vi "Multiple Class_Multiple State_Block Chain.vi"() -> ()   [LabVIEW 2021]
uses:
  Commander/Commander.lvclass
  C:/Program Files (x86)/Hyper State Machine Framework/SSW_Hyper_State_Machine.lvlibp/State_Machine_Class/Main_State_Machine/Hyper_State_Machine.lvclass
  C:/Program Files (x86)/Hyper State Machine Framework/SSW_Hyper_State_Machine.lvlibp/State_Interface/State_Interface.lvclass
  Common_State/Common_State.lvclass
  Image_Acquisition/Image_Acquisition.lvclass
  Motion_Control/Motion_Control.lvclass
  Data_Logging/Data_Logging.lvclass
  DIO/DIO.lvclass
  C:/Program Files (x86)/Hyper State Machine Framework/SSW_Hyper_State_Machine.lvlibp/State_Machine_Class/State_Machine_Module.llb/State Machine.ctl
  C:/Program Files (x86)/Hyper State Machine Framework/SSW_Hyper_State_Machine.lvlibp/State_Machine_Class/State_Machine_Module.llb/Lock_Unlock.ctl
  C:/Program Files (x86)/Hyper State Machine Framework/SSW_Hyper_State_Machine.lvlibp/State_Machine_Class/State_Machine_Module.llb/Iterval.ctl
  C:/Program Files (x86)/Hyper State Machine Framework/SSW_Hyper_State_Machine.lvlibp/State_Machine_Class/State_Machine_Module.llb/Time_Out.ctl
  <vilib>/numeric/Random Number (Range) DBL.vi
  <vilib>/Utility/High Resolution Relative Seconds.vi
  C:/Program Files (x86)/Hyper State Machine Framework/SSW_Hyper_State_Machine.lvlibp
panel:
  out "Child_State#":u32
  out "Activate":bool
  out "Lamp":bool
  out "Current_Pos":dbl caption="mm"
  in  "EMO":bool
  out "Product ID":string
  in  "Activate_Code(Blank for 30 min Trial)":string="ROeInPkJ3DxAXwEgzbbW2XA0t1jaS1URlS9jikesQMED6VfU"
  out "Heart_Rate":bool
  out "Heart rate(s)":dbl format="%#_6p"
  out "Execute rate(Hz)":dbl format="%#_6p"
  out "Base Class_Time_Act":bool
  out "Base Class_Elapsed Time(s)":dbl format="%#_6p"
  out "Base Class":bool=TRUE
  out "Base Class_Remaining(s)":dbl format="%#_6p"
  out "Base Class Progress":dbl(slide) scale=0.0..10.0
  in  "Base Class":dbl=10.0 max=1000.0 format="%#_13p"
  out "Base Class":string
  out "Base Class_Active":bool
  in  "Action Manager":T1(ring)
  out "Common":bool=TRUE
  out "Common_State":string
  out "Common_Time_Act":bool
  out "Common_Elapsed Time(s)":dbl format="%#_6p"
  out "Common_State Progress":dbl(slide) scale=0.0..5.0
  in  "Common_State_Interval":dbl=5.0 max=1000.0 format="%#_13p"
  out "Common_State_Active":bool
  out "Common_State_Remaining(s)":dbl format="%#_6p"
  out "Data Logging Progress":dbl(slide) scale=0.0..3.0
  out "DIO Progress":dbl(slide) scale=0.0..0.01
  out "Motion Control Progress":dbl(slide) scale=0.0..0.5
  out "Image Acquisition Progress":dbl(slide) scale=0.0..0.01
  out "Commander Progress":dbl(slide)=-1.0 scale=0.0..1.0
  out "Data_Logging":bool=TRUE
  out "Data Logging":string
  out "Data_Logging_Time_Act":bool
  out "Data_Logging_Elapsed Time(s)":dbl format="%#_6p"
  out "DIO":bool=TRUE
  out "DIO":string
  out "DIO_Time_Act":bool
  out "DIO_Elapsed Time(s)":dbl format="%#_6p"
  out "Motion_Control":bool=TRUE
  out "Motion_Control":string
  out "Motion_Control_Time_Act":bool
  out "Motion_Control_Elapsed Time(s)":dbl format="%#_6p"
  in  "Data Logging":dbl=3.0 max=1000.0 format="%#_13p"
  out "Data Logging_Active":bool
  out "Data Logging_Remaining(s)":dbl format="%#_6p"
  in  "DIO_Interval":dbl=0.01 max=1000.0 format="%#_13p"
  in  "Motion_Control_Interval":dbl=0.5 max=1000.0 format="%#_13p"
  out "Motion Control_Act":bool
  out "DIO_Act":bool
  out "DIO_Remaining(s)":dbl format="%#_6p"
  out "Motion_Control_Remaining(s)":dbl format="%#_6p"
  in  "Image Acquisition_Interval":dbl=0.01 max=1000.0 format="%#_13p"
  in  "Commander_Interval":dbl max=1000.0 format="%#_13p"
  in  "System_Wait_Time":dbl=0.025 format="%#_13p"
  out "Commander_Active":bool
  out "Image Acquisition_Act":bool
  out "Image Acquisition_Remaining(s)":dbl format="%#_6p"
  out "Commander_Remaining(s)":dbl format="%#_6p"
  out "Image Acquisition":bool=TRUE
  out "Image Acquisition":string
  out "Commander":bool=TRUE
  out "Image Acquisition_Time_Act":bool
  out "Image Acquisition_Elapsed Time(s)":dbl format="%#_6p"
  out "Commander":string
  out "State1_Time_Act":bool
  out "Commander_Elapsed Time(s)":dbl format="%#_6p"
  in  "Stop":bool
  # "Note : Each State is Waiting Until Commader State Finished on \"Interval_Delay\" and then Unlock"
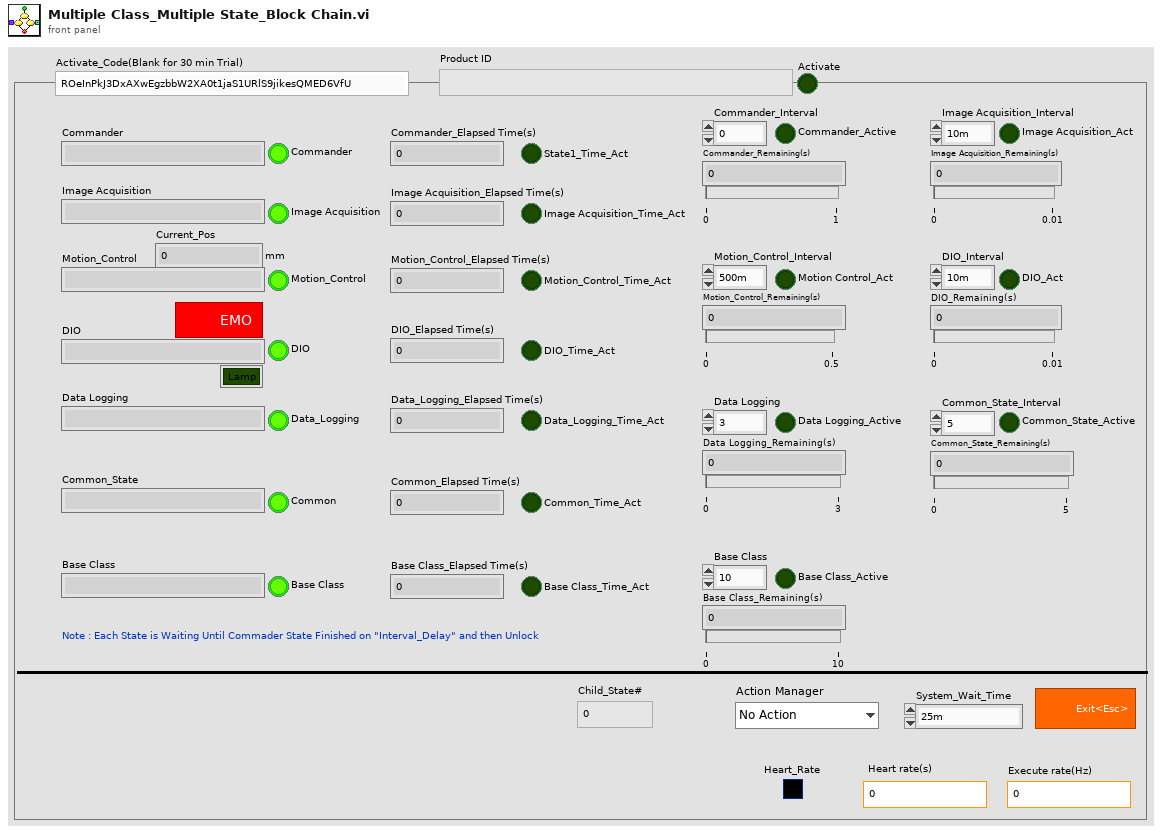
[diagram p1: front panel]
types:
  T1 = enum16{"No Action", "Init", "Lock", "Unlock", "Release"}
  T2 = typedef "SSW_Hyper_State_Machine.lvlibp/State Machine.ctl" = cluster{"Command":string, "Data":variant}
  T3 = typedef "SSW_Hyper_State_Machine.lvlibp/Time_Out.ctl" = cluster{"Enable(True)":bool, "Time Out_State Name":string, "Time Target (1s)":dbl, "Time Out_Reply Message_State":string}
  T4 = typedef "SSW_Hyper_State_Machine.lvlibp/Lock_Unlock.ctl" = cluster{"Action_Mode (Get)":enum16{"Set", "Get"}, "Action_Set (False)":bool, "State_In (Wait)":string}
  T5 = typedef "SSW_Hyper_State_Machine.lvlibp/Iterval.ctl" = cluster{"Delay(s)":dbl, "State (Interval_Delay)":string}
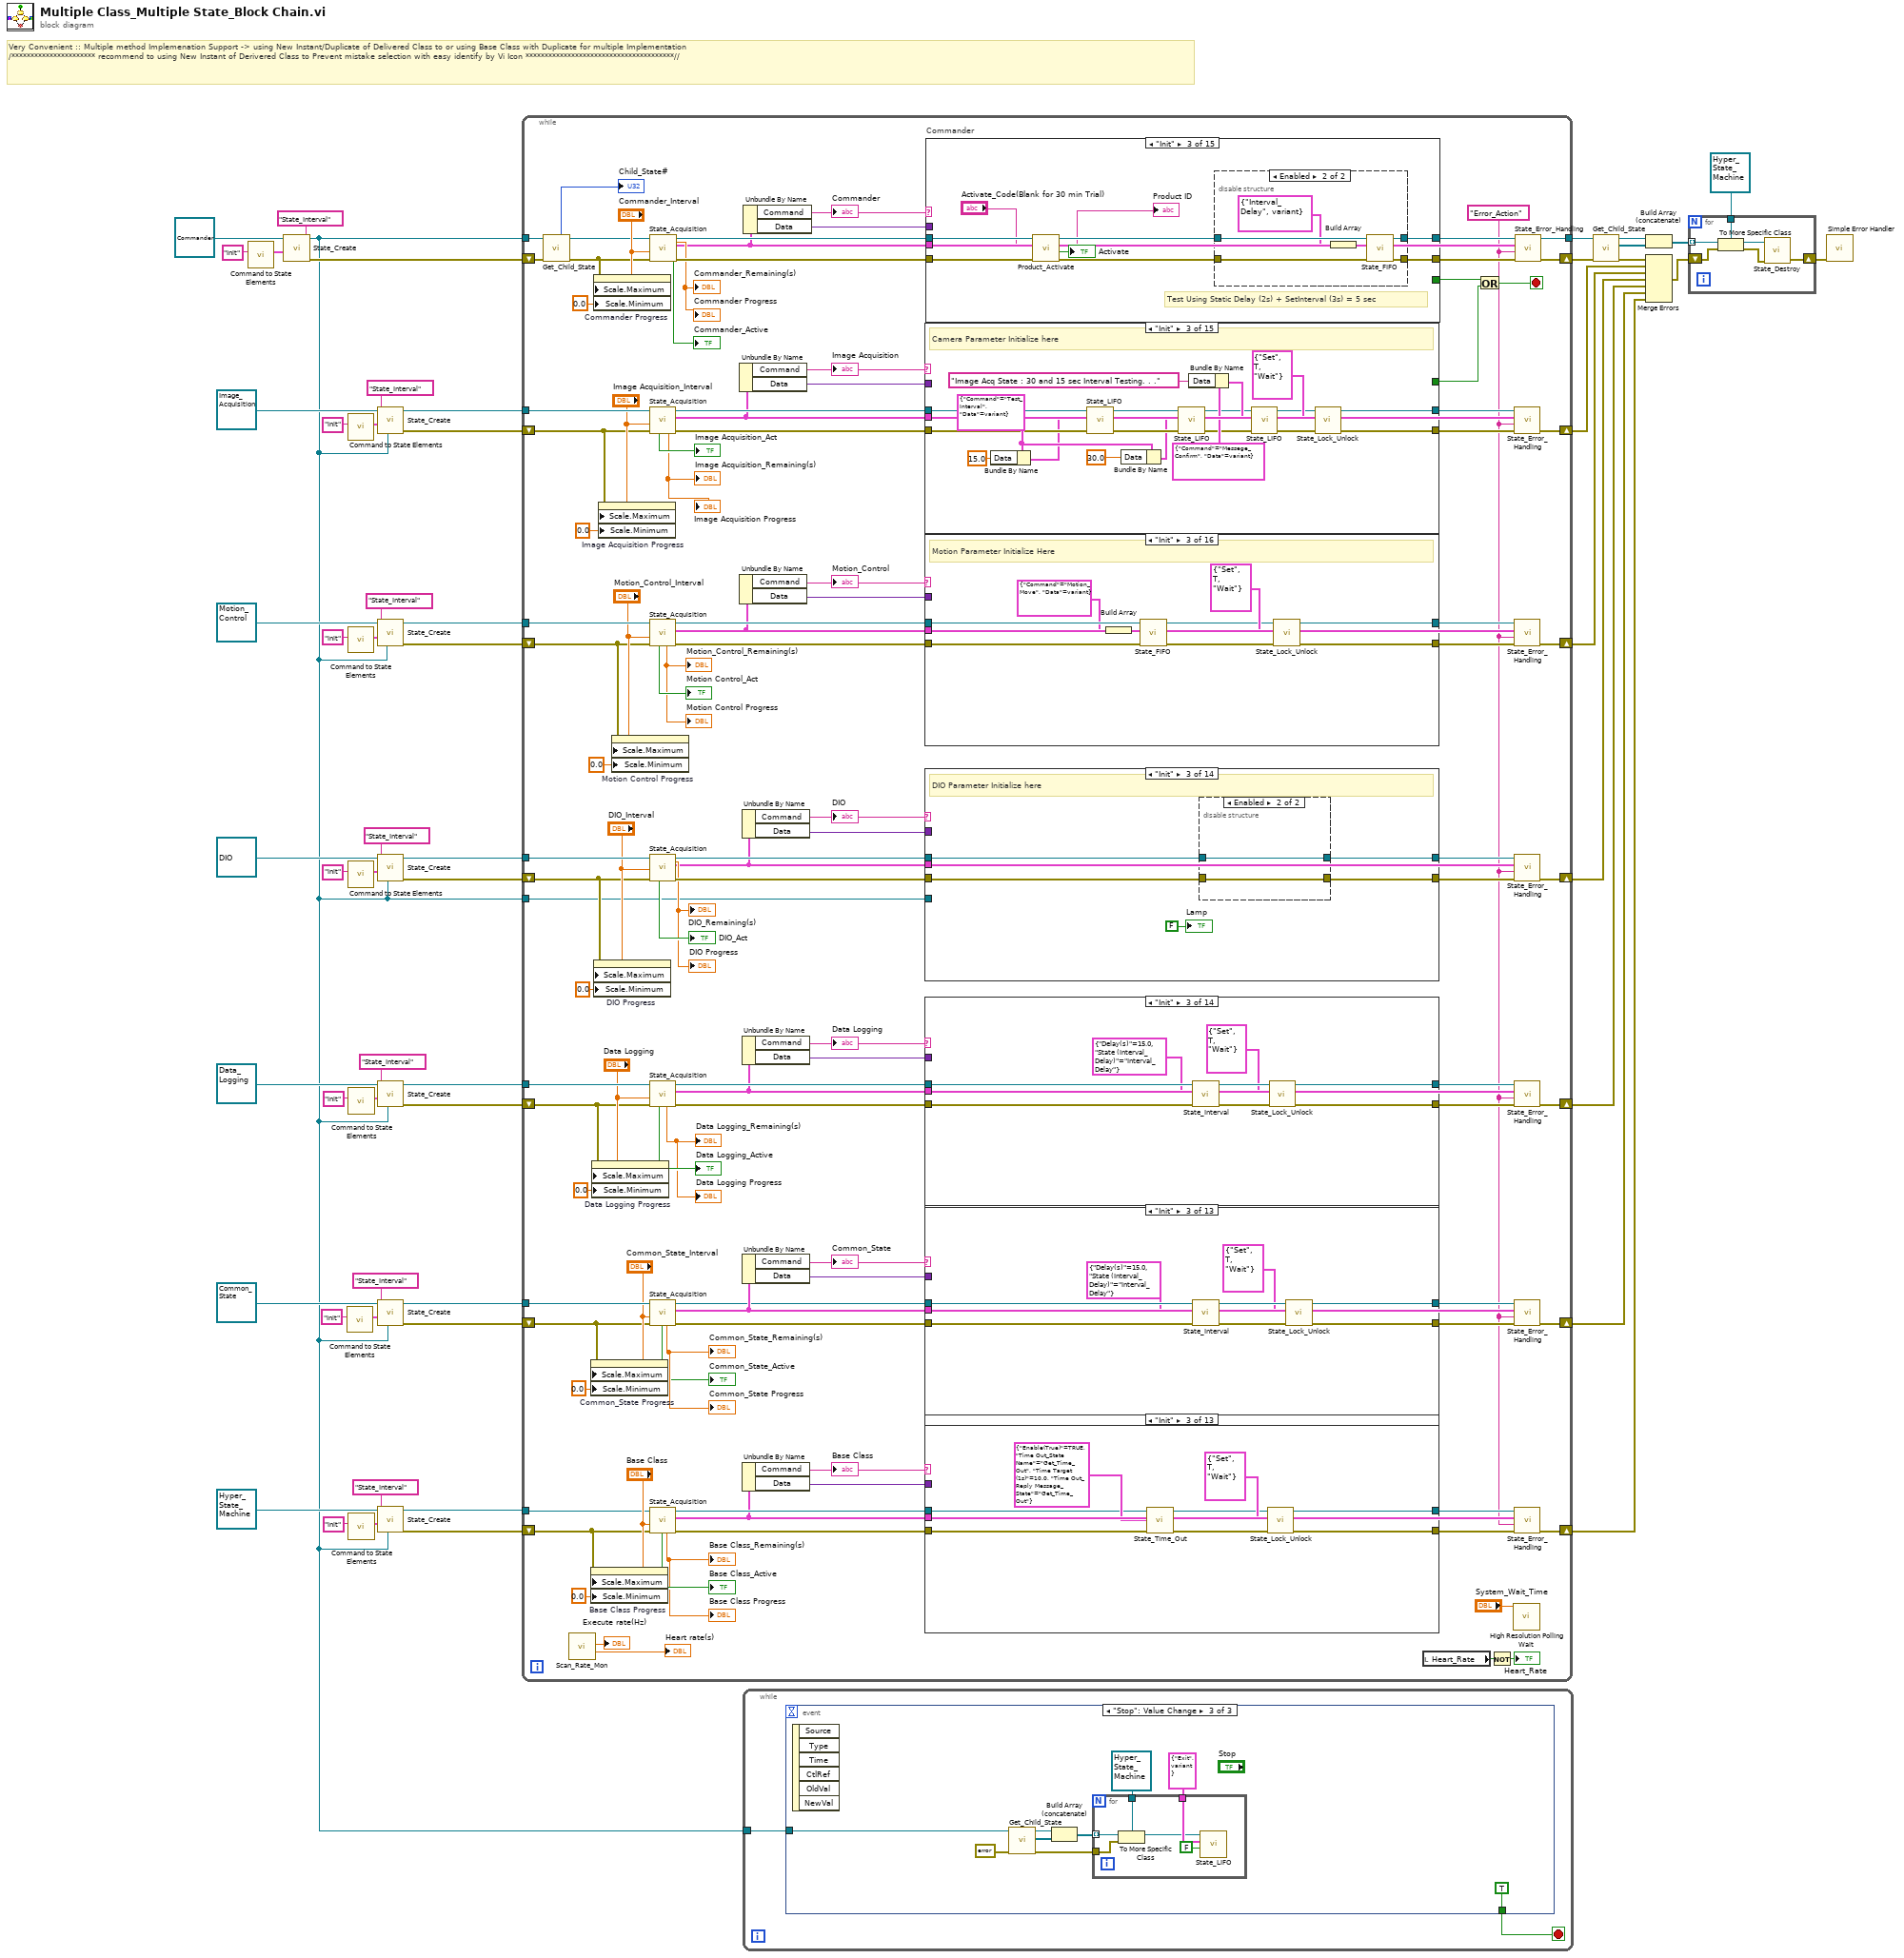
[diagram p0: block diagram]
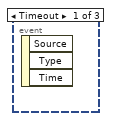
[diagram p2: hidden frame]
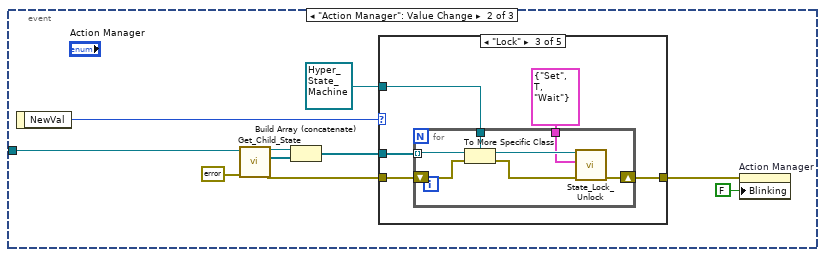
[diagram p3: hidden frame]
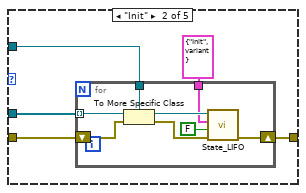
[diagram p5: hidden frame]
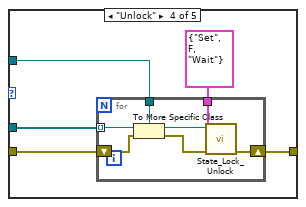
[diagram p6: hidden frame]
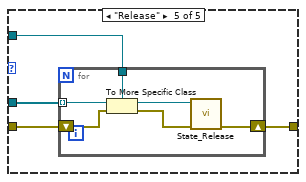
[diagram p7: hidden frame]
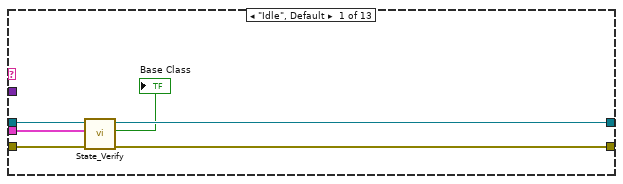
[diagram p8: hidden frame]
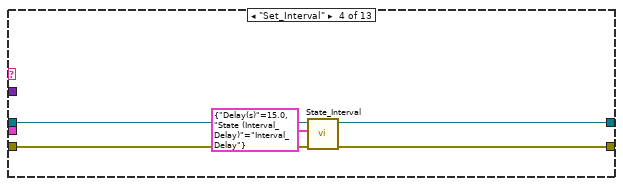
[diagram p10: hidden frame]
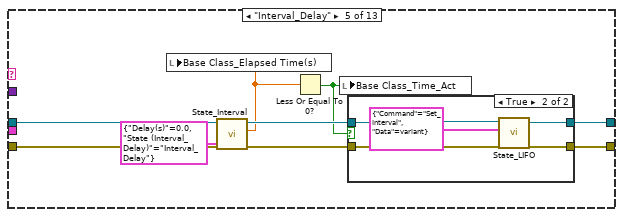
[diagram p11: hidden frame]
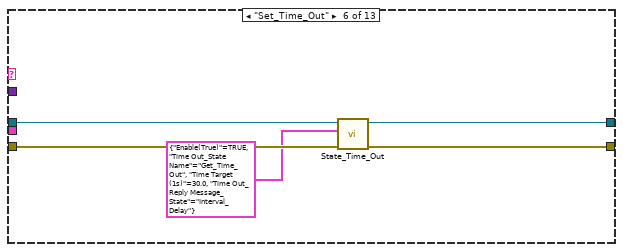
[diagram p13: hidden frame]
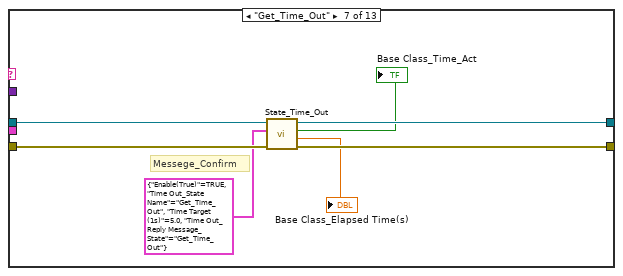
[diagram p14: hidden frame]
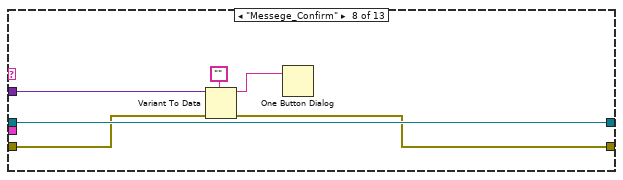
[diagram p15: hidden frame]
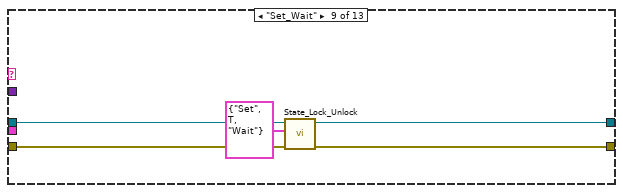
[diagram p16: hidden frame]
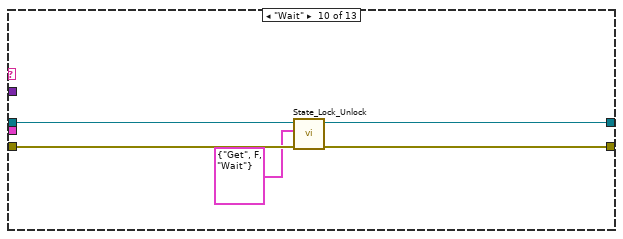
[diagram p17: hidden frame]
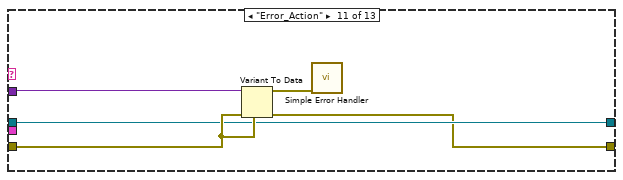
[diagram p18: hidden frame]
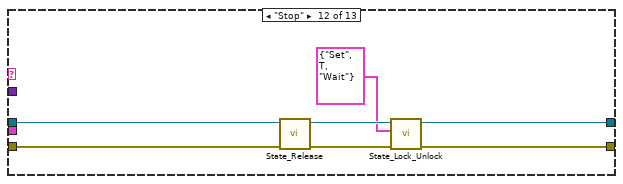
[diagram p19: hidden frame]
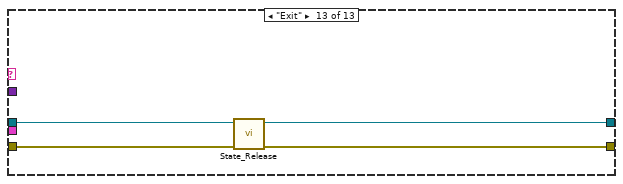
[diagram p20: hidden frame]
diagram:
  # "Very Convenient :: Multiple method Implemenation Support -> using New Instant/Duplicate of Delivered Class to or using Base Class with Duplicate for multiple Implementation\n/********************** recommend to using New Instant of Derivered Class to Prevent mistake selection with easy identify by Vi Icon ***************************************//"
  n1 = call "Command to State Elements.vi"("Command"="Init") -> ("Command to State Elements"=w40:T2)  [unwired: 10 in]
  n2 = call-dynamic "State_Create.vi"("Init_State(Option)"=w40, "State_Interval_Name"="State_Interval" ("Core_Interval_Name(State_Interval)"), "State_Machine_Class in"=refnum<class "Commander.lvclass"> refnum ("Commander.lvclass")) -> ("error out"=w57:errorcluster, "State_Machine_Class out"=w16:refnum<class "Commander.lvclass">)  [unwired: 6 in, 1 out]
  n3 = call "Command to State Elements.vi"("Command"="Init") -> ("Command to State Elements"=w32:T2)  [unwired: 10 in]
  n4 = call "Command to State Elements.vi"("Command"="Init") -> ("Command to State Elements"=w42:T2)  [unwired: 10 in]
  n5 = call "Command to State Elements.vi"("Command"="Init") -> ("Command to State Elements"=w38:T2)  [unwired: 10 in]
  n6 = call "Command to State Elements.vi"("Command"="Init") -> ("Command to State Elements"=w36:T2)  [unwired: 10 in]
  n7 = call "Command to State Elements.vi"("Command"="Init") -> ("Command to State Elements"=w34:T2)  [unwired: 10 in]
  n8 = call "Command to State Elements.vi"("Command"="Init") -> ("Command to State Elements"=w30:T2)  [unwired: 10 in]
  n9 = call-dynamic "State_Create.vi"("Block_Chain"=w16, "Init_State(Option)"=w42, "State_Interval_Name"="State_Interval" ("Core_Interval_Name(State_Interval)"), "State_Machine_Class in"=refnum<class "Image_Acquisition.lvclass"> refnum ("Image_Acquisition.lvclass")) -> ("error out"=w56:errorcluster, "State_Machine_Class out"=w22:refnum<class "Image_Acquisition.lvclass">)  [unwired: 5 in, 1 out]
  n10 = call-dynamic "State_Create.vi"("Block_Chain"=w16, "Init_State(Option)"=w38, "State_Interval_Name"="State_Interval" ("Core_Interval_Name(State_Interval)"), "State_Machine_Class in"=refnum<class "Motion_Control.lvclass"> refnum ("Motion_Control.lvclass")) -> ("error out"=w51:errorcluster, "State_Machine_Class out"=w21:refnum<class "Motion_Control.lvclass">)  [unwired: 5 in, 1 out]
  n11 = call-dynamic "State_Create.vi"("Block_Chain"=w16, "Init_State(Option)"=w36, "State_Interval_Name"="State_Interval" ("Core_Interval_Name(State_Interval)"), "State_Machine_Class in"=refnum<class "DIO.lvclass"> refnum ("DIO.lvclass")) -> ("error out"=w50:errorcluster, "State_Machine_Class out"=w20:refnum<class "DIO.lvclass">)  [unwired: 5 in, 1 out]
  n12 = call-dynamic "State_Create.vi"("Block_Chain"=w16, "Init_State(Option)"=w34, "State_Interval_Name"="State_Interval" ("Core_Interval_Name(State_Interval)"), "State_Machine_Class in"=refnum<class "Data_Logging.lvclass"> refnum ("Data_Logging.lvclass")) -> ("error out"=w49:errorcluster, "State_Machine_Class out"=w19:refnum<class "Data_Logging.lvclass">)  [unwired: 5 in, 1 out]
  n13 = call-dynamic "State_Create.vi"("Block_Chain"=w16, "Init_State(Option)"=w32, "State_Interval_Name"="State_Interval" ("Core_Interval_Name(State_Interval)"), "State_Machine_Class in"=refnum<class "Common_State.lvclass"> refnum ("Common_State.lvclass")) -> ("error out"=w47:errorcluster, "State_Machine_Class out"=w18:refnum<class "Common_State.lvclass">)  [unwired: 5 in, 1 out]
  n14 = call-dynamic "State_Create.vi"("Parent_State"=w16, "Init_State(Option)"=w30, "State_Interval_Name"="State_Interval" ("Core_Interval_Name(State_Interval)"), "State_Machine_Class in"=refnum<class "Hyper_State_Machine.lvclass"> refnum ("SSW_Hyper_State_Machine.lvlibp:Hyper_State_Machine.lvclass")) -> ("error out"=w44:errorcluster, "State_Machine_Class out"=w17:refnum<class "Hyper_State_Machine.lvclass">)  [unwired: 5 in, 1 out]
  n15 = while {
    tunnel: w16 -> [w62]
    shift-right: [w163] -> w14
    shift-left: w57 -> [w61]
    tunnel: [w162] -> w15
    tunnel: w22 -> [w158]
    shift-right: [w157] -> w6
    shift-left: w56 -> [w69]
    tunnel: w21 -> [w134]
    tunnel: w20 -> [w133]
    tunnel: w19 -> [w132]
    shift-right: [w131] -> w5
    shift-left: w51 -> [w68]
    shift-right: [w130] -> w4
    shift-left: w50 -> [w67]
    shift-right: [w129] -> w3
    shift-left: w49 -> [w66]
    tunnel: w18 -> [w108]
    shift-right: [w107] -> w2
    shift-left: w47 -> [w65]
    shift-right: [w77] -> w1
    shift-left: w44 -> [w64]
    tunnel: w17 -> [w81]
    tunnel: w16 -> [w63]
    stop <- w155 stop-if-true
    w76 = "Error_Action" ("State_Error_Handling")
    n16 = call-dynamic "Get_Child_State.vi"("error in (no error)"=w61, "Hyper_State_Machine in"=w62) -> ("error out"=w60:errorcluster, "Hyper_State_Machine out"=w59:refnum<class "Commander.lvclass">, "Child_State#"=→"Child_State#":u32)  [unwired: 5 in, 2 out]
    n17 = call "Scan_Rate_Mon.vi"() -> ("Heart rate(s)"=→"Heart rate(s)":dbl, "Execute rate(Hz)"=→"Execute rate(Hz)":dbl)
    n18 = property on="Common_State Progress" class="Slide (strict)"(error in=w65, "Scale.Maximum"="Common_State_Interval", "Scale.Minimum"=0.0 ("Scale.Range:Minimum")) -> ()  [unwired: 1 in, 2 out]
    n19 = property on="Base Class Progress" class="Slide (strict)"(error in=w64, "Scale.Maximum"="Base Class", "Scale.Minimum"=0.0 ("Scale.Range:Minimum")) -> ()  [unwired: 1 in, 2 out]
    n20 = property on="Data Logging Progress" class="Slide (strict)"(error in=w66, "Scale.Maximum"="Data Logging", "Scale.Minimum"=0.0 ("Scale.Range:Minimum")) -> ()  [unwired: 1 in, 2 out]
    n21 = property on="Commander Progress" class="Slide (strict)"(error in=w60, "Scale.Maximum"="Commander_Interval", "Scale.Minimum"=0.0 ("Scale.Range:Minimum")) -> ()  [unwired: 1 in, 2 out]
    n22 = property on="DIO Progress" class="Slide (strict)"(error in=w67, "Scale.Maximum"="DIO_Interval", "Scale.Minimum"=0.0 ("Scale.Range:Minimum")) -> ()  [unwired: 1 in, 2 out]
    n23 = property on="Image Acquisition Progress" class="Slide (strict)"(error in=w69, "Scale.Maximum"="Image Acquisition_Interval", "Scale.Minimum"=0.0 ("Scale.Range:Minimum")) -> ()  [unwired: 1 in, 2 out]
    n24 = property on="Motion Control Progress" class="Slide (strict)"(error in=w68, "Scale.Maximum"="Motion_Control_Interval", "Scale.Minimum"=0.0 ("Scale.Range:Minimum")) -> ()  [unwired: 1 in, 2 out]
    n25 = call-dynamic "State_Acquisition.vi"("error in (no error)"=w69, "State_Interval_Time(s)"="Image Acquisition_Interval", "Main_Machine_State_Class in"=w158) -> ("error out"=w161:errorcluster, "State"=w94:T2, "Main_Machine_State_Class out"=w156:refnum<class "Image_Acquisition.lvclass">, "Remaining(ms)"=→"Image Acquisition_Remaining(s)" →"Image Acquisition Progress":dbl, "Current_State_Active"=→"Image Acquisition_Act":bool)  [unwired: 2 in, 2 out]
    n26 = call-dynamic "State_Acquisition.vi"("error in (no error)"=w68, "State_Interval_Time(s)"="Motion_Control_Interval", "Main_Machine_State_Class in"=w134) -> ("error out"=w136:errorcluster, "State"=w93:T2, "Main_Machine_State_Class out"=w137:refnum<class "Motion_Control.lvclass">, "Remaining(ms)"=→"Motion_Control_Remaining(s)" →"Motion Control Progress":dbl, "Current_State_Active"=→"Motion Control_Act":bool)  [unwired: 2 in, 2 out]
    n27 = call-dynamic "State_Acquisition.vi"("error in (no error)"=w67, "State_Interval_Time(s)"="DIO_Interval", "Main_Machine_State_Class in"=w133) -> ("error out"=w143:errorcluster, "State"=w92:T2, "Main_Machine_State_Class out"=w144:refnum<class "DIO.lvclass">, "Remaining(ms)"=→"DIO_Remaining(s)" →"DIO Progress":dbl, "Current_State_Active"=→"DIO_Act":bool)  [unwired: 2 in, 2 out]
    n28 = call-dynamic "State_Acquisition.vi"("error in (no error)"=w66, "State_Interval_Time(s)"="Data Logging", "Main_Machine_State_Class in"=w132) -> ("error out"=w145:errorcluster, "State"=w91:T2, "Main_Machine_State_Class out"=w146:refnum<class "Data_Logging.lvclass">, "Remaining(ms)"=→"Data Logging_Remaining(s)" →"Data Logging Progress":dbl, "Current_State_Active"=→"Data Logging_Active":bool)  [unwired: 2 in, 2 out]
    n29 = call-dynamic "State_Acquisition.vi"("error in (no error)"=w65, "State_Interval_Time(s)"="Common_State_Interval", "Main_Machine_State_Class in"=w108) -> ("error out"=w110:errorcluster, "State"=w90:T2, "Main_Machine_State_Class out"=w75:refnum<class "Common_State.lvclass">, "Remaining(ms)"=→"Common_State_Remaining(s)" →"Common_State Progress":dbl, "Current_State_Active"=→"Common_State_Active":bool)  [unwired: 2 in, 2 out]
    n30 = call-dynamic "State_Acquisition.vi"("error in (no error)"=w64, "State_Interval_Time(s)"="Base Class", "Main_Machine_State_Class in"=w81) -> ("error out"=w82:errorcluster, "State"=w79:T2, "Main_Machine_State_Class out"=w83:refnum<class "Hyper_State_Machine.lvclass">, "Remaining(ms)"=→"Base Class_Remaining(s)" →"Base Class Progress":dbl, "Current_State_Active"=→"Base Class_Active":bool)  [unwired: 2 in, 2 out]
    n31 = call-dynamic "State_Acquisition.vi"("error in (no error)"=w60, "State_Interval_Time(s)"="Commander_Interval", "Main_Machine_State_Class in"=w59) -> ("error out"=w165:errorcluster, "State"=w95:T2, "Main_Machine_State_Class out"=w166:refnum<class "Commander.lvclass">, "Remaining(ms)"=→"Commander_Remaining(s)" →"Commander Progress":dbl, "Current_State_Active"=→"Commander_Active":bool)  [unwired: 2 in, 2 out]
    n32 = Unbundle By Name(w94) -> ("Command"=w159:string, "Data"=w160:variant)
    "Image Acquisition" <- w159
    n33 = Unbundle By Name(w93) -> ("Command"=w123:string, "Data"=w149:variant)
    "Motion_Control" <- w123
    n34 = Unbundle By Name(w92) -> ("Command"=w124:string, "Data"=w148:variant)
    "DIO" <- w124
    n35 = Unbundle By Name(w91) -> ("Command"=w125:string, "Data"=w147:variant)
    "Data Logging" <- w125
    n36 = Unbundle By Name(w90) -> ("Command"=w104:string, "Data"=w109:variant)
    "Common_State" <- w104
    n37 = Unbundle By Name(w79) -> ("Command"=w87:string, "Data"=w84:variant)
    "Base Class" <- w87
    n38 = Unbundle By Name(w95) -> ("Command"=w169:string, "Data"=w168:variant)
    "Commander" <- w169
    n39 = case shown="\"Init\"" w159 {
      selector: w159 -> [_ _ _ w659 _ _ _ _ _ _ _ _ _ _ _]
      tunnel: w160 -> [_ _ _ _ _ w674 _ _ _ w723 _ _ w737 _ _]
      tunnel: w156 -> [w635 w637 w645 w664 w669 w679 w692 w710 w717 w721 w728 w733 w734 w745 w750]
      tunnel: w161 -> [w634 w636 w640 w663 w668 w670 w691 w709 w716 w720 w727 w732 w736 w744 w749]
      tunnel: [w628 w637 w653 w662 w667 w678 w687 w708 w715 w721 w726 w731 w734 w740 w748] -> w151
      tunnel: [w627 w636 w652 w661 w666 w677 w686 w707 w714 w719 w725 w730 w735 w739 w747] -> w150
      tunnel: w94 -> [w633 _ _ _ _ _ _ _ _ _ _ _ _ _ _]
      tunnel: [_ _ _ _ _ _ _ _ _ _ _ _ _ _ TRUE] -> w154
      frame "Idle", Default {
        n40 = call-dynamic "State_Verify.vi"("error in (no error)"=w634, "State(Idle)"=w633, "State_Machine_Class in"=w635) -> ("error out"=w630:errorcluster, "Active"=→"Image Acquisition":bool, "State_Machine_Class out"=w631:refnum<class "Image_Acquisition.lvclass">)  [unwired: 6 in]
        n41 = Build Array(T2 {"Command"="Image_Acquisition", "Data"=variant} ("State")) -> (w626:T2[])
        n42 = call-dynamic "State_FIFO.vi"("error in (no error)"=w630, "State Machine[]"=w626, "State_Machine_Class in"=w631) -> ("error out"=w627:errorcluster, "State_Machine_Class out"=w628:refnum<class "Image_Acquisition.lvclass">)  [unwired: 7 in]
      }
      frame "State_Interval" {
      }
      frame "Init" {
        w648 = T2 {"Command"="Test_Interval", "Data"=variant} ("State Machine")
        # "Camera Parameter Initialize here"
        n43 = Bundle By Name(cluster=w648, "Data"=15.0) -> (w639:T2)
        n44 = call-dynamic "State_LIFO.vi"("error in (no error)"=w640, "State Machine"=w639, "State_Machine_Class in"=w645) -> ("error out"=w641:errorcluster, "State_Machine_Class out"=w644:refnum<class "Image_Acquisition.lvclass">)  [unwired: 7 in]
        n45 = Bundle By Name(cluster=w648, "Data"=30.0) -> (w638:T2)
        n46 = call-dynamic "State_LIFO.vi"("error in (no error)"=w641, "State Machine"=w638, "State_Machine_Class in"=w644) -> ("error out"=w642:errorcluster, "State_Machine_Class out"=w643:refnum<class "Image_Acquisition.lvclass">)  [unwired: 7 in]
        n47 = Bundle By Name(cluster=T2 {"Command"="Messege_Confirm", "Data"=variant} ("State Machine"), "Data"="Image Acq State : 30 and 15 sec Interval Testing. . .") -> (w650:T2)
        n48 = call-dynamic "State_LIFO.vi"("error in (no error)"=w642, "State Machine"=w650, "State_Machine_Class in"=w643) -> ("error out"=w654:errorcluster, "State_Machine_Class out"=w655:refnum<class "Image_Acquisition.lvclass">)  [unwired: 7 in]
        n49 = call-dynamic "State_Lock_Unlock.vi"("error in (no error)"=w654, "Parameter"=T4 {"Action_Mode (Get)"=enum."Set", "Action_Set (False)"=TRUE, "State_In (Wait)"="Wait"}, "State_Machine_Class in"=w655) -> ("error out"=w652:errorcluster, "State_Machine_Class out"=w653:refnum<class "Image_Acquisition.lvclass">)  [unwired: 6 in, 1 out]
      }
      frame "Image_Acquisition" {
        (unwired) T5 {"Delay(s)"=5.0, "State (Interval_Delay)"="Image_Acquisition"} ("Parameter")
        # "Simple handling with specify name"
        # "Dynamic handling Name for Waiting Demo"
        # "Image Acquisition Function Here"
        n50 = Bundle By Name(cluster=T5 {"Delay(s)"=5.0, "State (Interval_Delay)"=""} ("Parameter"), "State (Interval_Delay)"=w659) -> (w658:T5)
        n51 = call-dynamic "State_Interval.vi"("error in (no error)"=w663, "Parameter"=w658, "State_Machine_Class in"=w664) -> ("error out"=w661:errorcluster, "Elapsed Time(s)"=w657:dbl, "State_Machine_Class out"=w662:refnum<class "Image_Acquisition.lvclass">)  [unwired: 6 in]
        n52 = local write "Image Acquisition_Elapsed Time(s)"(w657) -> ()
      }
      frame "Set_Interval" {
        n53 = call-dynamic "State_Interval.vi"("error in (no error)"=w668, "Parameter"=T5 {"Delay(s)"=15.0, "State (Interval_Delay)"="Interval_Delay"}, "State_Machine_Class in"=w669) -> ("error out"=w666:errorcluster, "State_Machine_Class out"=w667:refnum<class "Image_Acquisition.lvclass">)  [unwired: 6 in, 1 out]
      }
      frame "Test_Interval" {
        n54 = Variant To Data(error in=w670, type=0.0 ("Delay(s)"), Variant=w674) -> (data=w672:dbl)  [unwired: 1 out]
        n55 = Bundle By Name(cluster=T5 {"Delay(s)"=0.0, "State (Interval_Delay)"="Test_Interval"} ("Parameter"), "Delay(s)"=w672) -> (w671:T5)
        n56 = call-dynamic "State_Interval.vi"("error in (no error)"=w670, "Parameter"=w671, "State_Machine_Class in"=w679) -> ("error out"=w677:errorcluster, "Elapsed Time(s)"=w676:dbl, "State_Machine_Class out"=w678:refnum<class "Image_Acquisition.lvclass">)  [unwired: 6 in]
        n57 = local write "Image Acquisition_Elapsed Time(s)"(w676) -> ()
      }
      frame "Interval_Delay" {
        n58 = call-dynamic "State_Interval.vi"("error in (no error)"=w691, "Parameter"=T5 {"Delay(s)"=0.0, "State (Interval_Delay)"="Interval_Delay"}, "State_Machine_Class in"=w692) -> ("error out"=w688:errorcluster, "Elapsed Time(s)"=w685:dbl, "State_Machine_Class out"=w689:refnum<class "Image_Acquisition.lvclass">)  [unwired: 6 in]
        "Image Acquisition_Elapsed Time(s)" <- w685
        n59 = Build Array(T2 {"Command"="Interval_Delay", "Data"=variant} ("State"), T2 {"Command"="Image_Acquisition", "Data"=variant} ("State")) -> (w681:T2[])
        n60 = Less Or Equal To 0?(x=w685) -> (x <= 0?=w690:bool)
        n61 = Reverse 1D Array(array=w681) -> (reversed array=w680:T2[])
        n62 = case shown="True" w690 {
          tunnel: w689 -> [w694 w699]
          tunnel: w688 -> [w693 w698]
          tunnel: [w694 w697] -> w687
          tunnel: [w693 w696] -> w686
          tunnel: w680 -> [_ w695]
          frame False {
          }
          frame True {
            n63 = for {
              shift-right: [w702] -> w697
              shift-left: w699 -> [w704]
              shift-right: [w701] -> w696
              shift-left: w698 -> [w703]
              tunnel: w695 -> [w700] mode=indexing
              n64 = call-dynamic "State_LIFO.vi"("error in (no error)"=w703, "State Machine"=w700, "State_Machine_Class in"=w704) -> ("error out"=w701:errorcluster, "State_Machine_Class out"=w702:refnum<class "Image_Acquisition.lvclass">)  [unwired: 7 in]
            }
          }
        }
        n65 = local write "Image Acquisition_Time_Act"(w690) -> ()
      }
      frame "Set_Time_Out" {
        n66 = call-dynamic "State_Time_Out.vi"("error in (no error)"=w709, "Parameter"=T3 {"Enable(True)"=TRUE, "Time Out_State Name"="Get_Time_Out", "Time Target (1s)"=30.0, "Time Out_Reply Message_State"="Messege_Confirm"}, "State_Machine_Class in"=w710) -> ("error out"=w707:errorcluster, "Timeout"=w706:bool, "State_Machine_Class out"=w708:refnum<class "Image_Acquisition.lvclass">)  [unwired: 5 in, 1 out]
        n67 = local write "Image Acquisition_Time_Act"(w706) -> ()
      }
      frame "Get_Time_Out" {
        # "Messege_Confirm"
        n68 = call-dynamic "State_Time_Out.vi"("error in (no error)"=w716, "Parameter"=T3 {"Enable(True)"=TRUE, "Time Out_State Name"="Get_Time_Out", "Time Target (1s)"=0.0, "Time Out_Reply Message_State"="Messege_Confirm"}, "State_Machine_Class in"=w717) -> ("error out"=w714:errorcluster, "Remaining Time (s)"=w713:dbl, "Timeout"=→"Image Acquisition_Time_Act":bool, "State_Machine_Class out"=w715:refnum<class "Image_Acquisition.lvclass">)  [unwired: 5 in]
        n69 = local write "Image Acquisition_Elapsed Time(s)"(w713) -> ()
      }
      frame "Messege_Confirm" {
        n70 = Variant To Data(error in=w720, type="", Variant=w723) -> (data=w718:string, error out=w719:errorcluster)
        n71 = One Button Dialog(message=w718) -> ()  [unwired: 1 in, 1 out]
      }
      frame "Set_Wait" {
        n72 = call-dynamic "State_Lock_Unlock.vi"("error in (no error)"=w727, "Parameter"=T4 {"Action_Mode (Get)"=enum."Set", "Action_Set (False)"=TRUE, "State_In (Wait)"="Wait"}, "State_Machine_Class in"=w728) -> ("error out"=w725:errorcluster, "State_Machine_Class out"=w726:refnum<class "Image_Acquisition.lvclass">)  [unwired: 6 in, 1 out]
      }
      frame "Wait" {
        n73 = call-dynamic "State_Lock_Unlock.vi"("error in (no error)"=w732, "Parameter"=T4 {"Action_Mode (Get)"=enum."Get", "Action_Set (False)"=FALSE, "State_In (Wait)"="Wait"}, "State_Machine_Class in"=w733) -> ("error out"=w730:errorcluster, "State_Machine_Class out"=w731:refnum<class "Image_Acquisition.lvclass">)  [unwired: 6 in, 1 out]
      }
      frame "Error_Action" {
        n74 = Variant To Data(error in=w736, type=w736, Variant=w737) -> (data=w738:errorcluster, error out=w735:errorcluster)
        n75 = call <vilib>:"Simple Error Handler.vi"("error in (no error)"=w738) -> ()  [unwired: 4 in, 5 out]
      }
      frame "Stop" {
        n76 = call-dynamic "State_Release.vi"("error in (no error)"=w744, "State_Machine_Class in"=w745) -> ("error out"=w742:errorcluster, "State_Machine_Class out"=w743:refnum<class "Image_Acquisition.lvclass">)  [unwired: 8 in]
        n77 = call-dynamic "State_Lock_Unlock.vi"("error in (no error)"=w742, "Parameter"=T4 {"Action_Mode (Get)"=enum."Set", "Action_Set (False)"=TRUE, "State_In (Wait)"="Wait"}, "State_Machine_Class in"=w743) -> ("error out"=w739:errorcluster, "State_Machine_Class out"=w740:refnum<class "Image_Acquisition.lvclass">)  [unwired: 6 in, 1 out]
      }
      frame "Exit" {
        n78 = call-dynamic "State_Release.vi"("error in (no error)"=w749, "State_Machine_Class in"=w750) -> ("error out"=w747:errorcluster, "State_Machine_Class out"=w748:refnum<class "Image_Acquisition.lvclass">)  [unwired: 8 in]
      }
    }
    n79 = case shown="\"Init\"" w123 {
      tunnel: w149 -> [_ _ _ _ _ _ _ _ _ _ w599 _ _ w612 _ _]
      tunnel: w137 -> [w535 w537 w543 w551 w556 w559 w564 w573 w586 w593 w597 w604 w609 w613 w621 w625]
      tunnel: w136 -> [w534 w536 w541 w550 w555 w558 w563 w572 w585 w592 w596 w603 w608 w611 w620 w624]
      tunnel: [w528 w537 w545 w549 w554 w559 w562 w569 w584 w591 w597 w602 w607 w613 w617 w623] -> w138
      tunnel: [w527 w536 w544 w548 w553 w558 w561 w568 w583 w590 w595 w601 w606 w610 w616 w622] -> w135
      tunnel: w93 -> [w533 _ _ _ _ _ _ _ _ _ _ _ _ _ _ _]
      frame "Idle", Default {
        n80 = call-dynamic "State_Verify.vi"("error in (no error)"=w534, "State(Idle)"=w533, "State_Machine_Class in"=w535) -> ("error out"=w530:errorcluster, "Active"=→"Motion_Control":bool, "State_Machine_Class out"=w531:refnum<class "Motion_Control.lvclass">)  [unwired: 6 in]
        n81 = Build Array(T2 {"Command"="Motion_Move", "Data"=variant} ("State")) -> (w526:T2[])
        n82 = call-dynamic "State_FIFO.vi"("error in (no error)"=w530, "State Machine[]"=w526, "State_Machine_Class in"=w531) -> ("error out"=w527:errorcluster, "State_Machine_Class out"=w528:refnum<class "Motion_Control.lvclass">)  [unwired: 7 in]
      }
      frame "State_Interval" {
        # "Handling Motion I/O or Cirtical Task Here"
      }
      frame "Init" {
        # "Motion Parameter Initialize Here"
        n83 = Build Array(T2 {"Command"="Motion_Move", "Data"=variant} ("State")) -> (w538:T2[])
        n84 = call-dynamic "State_FIFO.vi"("error in (no error)"=w541, "State Machine[]"=w538, "State_Machine_Class in"=w543) -> ("error out"=w540:errorcluster, "State_Machine_Class out"=w542:refnum<class "Motion_Control.lvclass">)  [unwired: 7 in]
        n85 = call-dynamic "State_Lock_Unlock.vi"("error in (no error)"=w540, "Parameter"=T4 {"Action_Mode (Get)"=enum."Set", "Action_Set (False)"=TRUE, "State_In (Wait)"="Wait"}, "State_Machine_Class in"=w542) -> ("error out"=w544:errorcluster, "State_Machine_Class out"=w545:refnum<class "Motion_Control.lvclass">)  [unwired: 6 in, 1 out]
      }
      frame "Motion_Move" {
        # "Motion Move Command here"
        n86 = call-dynamic "State_LIFO.vi"("error in (no error)"=w550, "State Machine"=T2 {"Command"="Motion_Request_Pos", "Data"=variant} ("State"), "State_Machine_Class in"=w551) -> ("error out"=w548:errorcluster, "State_Machine_Class out"=w549:refnum<class "Motion_Control.lvclass">)  [unwired: 7 in]
      }
      frame "Motion_Request_Pos" {
        # "Motion Query Position Command here"
        n87 = call-dynamic "State_LIFO.vi"("error in (no error)"=w555, "State Machine"=T2 {"Command"="Motion_Get_Pos", "Data"=variant} ("State"), "State_Machine_Class in"=w556) -> ("error out"=w553:errorcluster, "State_Machine_Class out"=w554:refnum<class "Motion_Control.lvclass">)  [unwired: 7 in]
      }
      frame "Motion_Get_Pos" {
        # "Motion Move Command here"
        n88 = call-poly <vilib>:"Random Number (Range).vi"() -> ("number"=→"Current_Pos":dbl)  [unwired: 11 in]
      }
      frame "Set_Interval" {
        n89 = call-dynamic "State_Interval.vi"("error in (no error)"=w563, "Parameter"=T5 {"Delay(s)"=15.0, "State (Interval_Delay)"="Interval_Delay"}, "State_Machine_Class in"=w564) -> ("error out"=w561:errorcluster, "State_Machine_Class out"=w562:refnum<class "Motion_Control.lvclass">)  [unwired: 6 in, 1 out]
      }
      frame "Interval_Delay" {
        n90 = call-dynamic "State_Interval.vi"("error in (no error)"=w572, "Parameter"=T5 {"Delay(s)"=0.0, "State (Interval_Delay)"="Interval_Delay"}, "State_Machine_Class in"=w573) -> ("error out"=w570:errorcluster, "Elapsed Time(s)"=w567:dbl, "State_Machine_Class out"=w571:refnum<class "Motion_Control.lvclass">)  [unwired: 6 in]
        n91 = local write "Motion_Control_Elapsed Time(s)"(w567) -> ()
        n92 = Less Or Equal To 0?(x=w567) -> (x <= 0?=w566:bool)
        n93 = local write "Motion_Control_Time_Act"(w566) -> ()
        n94 = case shown="True" w566 {
          tunnel: w571 -> [w575 w581]
          tunnel: w570 -> [w574 w580]
          tunnel: [w575 w579] -> w569
          tunnel: [w574 w578] -> w568
          frame False {
          }
          frame True {
            n95 = call-dynamic "State_LIFO.vi"("error in (no error)"=w580, "State_Interval(Enable)"=FALSE, "State Machine"=T2 {"Command"="Set_Interval", "Data"=variant} ("State"), "State_Machine_Class in"=w581) -> ("error out"=w578:errorcluster, "State_Machine_Class out"=w579:refnum<class "Motion_Control.lvclass">)  [unwired: 6 in]
          }
        }
      }
      frame "Set_Time_Out" {
        n96 = call-dynamic "State_Time_Out.vi"("error in (no error)"=w585, "Parameter"=T3 {"Enable(True)"=TRUE, "Time Out_State Name"="Get_Time_Out", "Time Target (1s)"=30.0, "Time Out_Reply Message_State"="Messege_Confirm"}, "State_Machine_Class in"=w586) -> ("error out"=w583:errorcluster, "State_Machine_Class out"=w584:refnum<class "Motion_Control.lvclass">)  [unwired: 5 in, 2 out]
      }
      frame "Get_Time_Out" {
        # "Messege_Confirm"
        n97 = call-dynamic "State_Time_Out.vi"("error in (no error)"=w592, "Parameter"=T3 {"Enable(True)"=TRUE, "Time Out_State Name"="Get_Time_Out", "Time Target (1s)"=0.0, "Time Out_Reply Message_State"="Messege_Confirm"}, "State_Machine_Class in"=w593) -> ("error out"=w590:errorcluster, "Remaining Time (s)"=→"Motion_Control_Elapsed Time(s)":dbl, "Timeout"=→"Motion_Control_Time_Act":bool, "State_Machine_Class out"=w591:refnum<class "Motion_Control.lvclass">)  [unwired: 5 in]
      }
      frame "Messege_Confirm" {
        n98 = Variant To Data(error in=w596, type="", Variant=w599) -> (data=w594:string, error out=w595:errorcluster)
        n99 = One Button Dialog(message=w594) -> ()  [unwired: 1 in, 1 out]
      }
      frame "Set_Wait" {
        n100 = call-dynamic "State_Lock_Unlock.vi"("error in (no error)"=w603, "Parameter"=T4 {"Action_Mode (Get)"=enum."Set", "Action_Set (False)"=TRUE, "State_In (Wait)"="Wait"}, "State_Machine_Class in"=w604) -> ("error out"=w601:errorcluster, "State_Machine_Class out"=w602:refnum<class "Motion_Control.lvclass">)  [unwired: 6 in, 1 out]
      }
      frame "Wait" {
        n101 = call-dynamic "State_Lock_Unlock.vi"("error in (no error)"=w608, "Parameter"=T4 {"Action_Mode (Get)"=enum."Get", "Action_Set (False)"=FALSE, "State_In (Wait)"="Wait"}, "State_Machine_Class in"=w609) -> ("error out"=w606:errorcluster, "State_Machine_Class out"=w607:refnum<class "Motion_Control.lvclass">)  [unwired: 6 in, 1 out]
      }
      frame "Error_Action" {
        n102 = Variant To Data(error in=w611, type=w611, Variant=w612) -> (data=w614:errorcluster, error out=w610:errorcluster)
        n103 = call <vilib>:"Simple Error Handler.vi"("error in (no error)"=w614) -> ()  [unwired: 4 in, 5 out]
      }
      frame "Stop" {
        n104 = call-dynamic "State_Release.vi"("error in (no error)"=w620, "State_Machine_Class in"=w621) -> ("error out"=w618:errorcluster, "State_Machine_Class out"=w619:refnum<class "Motion_Control.lvclass">)  [unwired: 8 in]
        n105 = call-dynamic "State_Lock_Unlock.vi"("error in (no error)"=w618, "Parameter"=T4 {"Action_Mode (Get)"=enum."Set", "Action_Set (False)"=TRUE, "State_In (Wait)"="Wait"}, "State_Machine_Class in"=w619) -> ("error out"=w616:errorcluster, "State_Machine_Class out"=w617:refnum<class "Motion_Control.lvclass">)  [unwired: 6 in, 1 out]
      }
      frame "Exit" {
        n106 = call-dynamic "State_Release.vi"("error in (no error)"=w624, "State_Machine_Class in"=w625) -> ("error out"=w622:errorcluster, "State_Machine_Class out"=w623:refnum<class "Motion_Control.lvclass">)  [unwired: 8 in]
      }
    }
    n107 = case shown="\"Init\"" w124 {
      tunnel: w148 -> [_ _ _ _ _ _ _ _ w496 _ _ w509 _ _]
      tunnel: w144 -> [w426 w433 w447 w462 w469 w474 w481 w487 w494 w501 w506 w507 w521 w525]
      tunnel: w143 -> [w425 _ w446 w461 w468 w473 w480 w486 w493 w500 w505 w510 w520 w524]
      tunnel: [w420 w433 w450 w460 w464 w472 w479 w485 w494 w499 w504 w507 w517 w523] -> w142
      tunnel: [w419 w427 w449 w459 w463 w471 w478 w484 w492 w498 w503 w508 w514 w522] -> w141
      tunnel: w92 -> [w424 _ _ _ _ _ _ _ _ _ _ _ _ _]
      tunnel: w63 -> [_ w430 _ _ _ _ _ _ _ _ _ _ _ _]
      frame "Idle", Default {
        # "Able to activate at \"Stae_Interval\""
        n108 = call-dynamic "State_Verify.vi"("error in (no error)"=w425, "State(Idle)"=w424, "State_Machine_Class in"=w426) -> ("error out"=w421:errorcluster, "Active"=→"DIO":bool, "State_Machine_Class out"=w422:refnum<class "DIO.lvclass">)  [unwired: 6 in]
        n109 = Build Array(T2 {"Command"="Lamp_Blinking", "Data"=variant} ("State")) -> (w417:T2[])
        n110 = call-dynamic "State_FIFO.vi"("error in (no error)"=w421, "State Machine[]"=w417, "State_Machine_Class in"=w422) -> ("error out"=w419:errorcluster, "State_Machine_Class out"=w420:refnum<class "DIO.lvclass">)  [unwired: 7 in]
      }
      frame "State_Interval" {
        # "Able to assign to Even to handling"
        # "Simulation of Emergency Signal , Pree to try (Can not Override State Lock if in Active)"
        # "Simulation of Emergency Signal"
        # "Every Cycle Time DIO Get Data Here"
        n111 = call-dynamic "Get_Child_State.vi"("Hyper_State_Machine in"=w430) -> ("error out"=w427:errorcluster, "Child_State"=w429:refnum<class "State_Interface.lvclass">[], "Hyper_State_Machine out"=w428:refnum<class "Commander.lvclass">)  [unwired: 6 in, 2 out]
        n112 = Build Array (concatenate)(w428, w429) -> (w431:refnum<class "State_Interface.lvclass">[])
        n113 = case shown="True" "EMO" {
          tunnel: w427 -> [_ w437]
          tunnel: w431 -> [_ w434]
          frame False {
          }
          frame True {
            n114 = for {
              shift-right: [w445] -> _
              shift-left: w437 -> [w439]
              tunnel: T2 {"Command"="Stop", "Data"=variant} ("State") -> [w443]
              tunnel: refnum<class "Hyper_State_Machine.lvclass"> refnum ("SSW_Hyper_State_Machine.lvlibp:Hyper_State_Machine.lvclass") -> [w442]
              tunnel: w434 -> [w440] mode=indexing
              n115 = To More Specific Class(target class=w442, reference=w440, error in=w439) -> (specific class reference=w441:refnum<class "Hyper_State_Machine.lvclass">, error out=w438:errorcluster)
              n116 = call-dynamic "State_LIFO.vi"("error in (no error)"=w438, "State_Interval(Enable)"=FALSE, "State Machine"=w443, "State_Machine_Class in"=w441) -> ("error out"=w445:errorcluster)  [unwired: 6 in, 1 out]
            }
          }
        }
      }
      frame "Init" {
        # "DIO Parameter Initialize here"
        n117 = disable-structure shown="Enabled" {
          disable-tunnel: [w455 w457] -> w450
          disable-tunnel: [w454 w456] -> w449
          disable-tunnel: w447 -> [w452 w457]
          disable-tunnel: w446 -> [w451 w456]
          frame Disabled {
            n118 = call-dynamic "State_Lock_Unlock.vi"("error in (no error)"=w451, "Parameter"=T4 {"Action_Mode (Get)"=enum."Set", "Action_Set (False)"=TRUE, "State_In (Wait)"="Wait"}, "State_Machine_Class in"=w452) -> ("error out"=w454:errorcluster, "State_Machine_Class out"=w455:refnum<class "DIO.lvclass">)  [unwired: 6 in, 1 out]
          }
          frame Enabled {
          }
        }
        "Lamp" <- FALSE ("Lamp")
      }
      frame "Set_Interval" {
        n119 = call-dynamic "State_Interval.vi"("error in (no error)"=w461, "Parameter"=T5 {"Delay(s)"=15.0, "State (Interval_Delay)"="Interval_Delay"}, "State_Machine_Class in"=w462) -> ("error out"=w459:errorcluster, "State_Machine_Class out"=w460:refnum<class "DIO.lvclass">)  [unwired: 6 in, 1 out]
      }
      frame "Interval_Delay" {
        n120 = call-dynamic "State_Interval.vi"("error in (no error)"=w468, "Parameter"=T5 {"Delay(s)"=0.0, "State (Interval_Delay)"="Interval_Delay"}, "State_Machine_Class in"=w469) -> ("error out"=w463:errorcluster, "Elapsed Time(s)"=w467:dbl, "State_Machine_Class out"=w464:refnum<class "DIO.lvclass">)  [unwired: 6 in]
        n121 = local write "DIO_Elapsed Time(s)"(w467) -> ()
        n122 = Less Or Equal To 0?(x=w467) -> (x <= 0?=w466:bool)
        n123 = local write "DIO_Time_Act"(w466) -> ()
      }
      frame "Set_Time_Out" {
        n124 = call-dynamic "State_Time_Out.vi"("error in (no error)"=w473, "Parameter"=T3 {"Enable(True)"=TRUE, "Time Out_State Name"="Get_Time_Out", "Time Target (1s)"=30.0, "Time Out_Reply Message_State"="Messege_Confirm"}, "State_Machine_Class in"=w474) -> ("error out"=w471:errorcluster, "State_Machine_Class out"=w472:refnum<class "DIO.lvclass">)  [unwired: 5 in, 2 out]
      }
      frame "Get_Time_Out" {
        # "Messege_Confirm"
        n125 = call-dynamic "State_Time_Out.vi"("error in (no error)"=w480, "Parameter"=T3 {"Enable(True)"=TRUE, "Time Out_State Name"="Get_Time_Out", "Time Target (1s)"=0.0, "Time Out_Reply Message_State"="Messege_Confirm"}, "State_Machine_Class in"=w481) -> ("error out"=w478:errorcluster, "Remaining Time (s)"=→"DIO_Elapsed Time(s)":dbl, "Timeout"=→"DIO_Time_Act":bool, "State_Machine_Class out"=w479:refnum<class "DIO.lvclass">)  [unwired: 5 in]
      }
      frame "Lamp_Blinking" {
        n126 = call-dynamic "State_Interval.vi"("error in (no error)"=w486, "Parameter"=T5 {"Delay(s)"=0.25, "State (Interval_Delay)"="Lamp_Blinking"}, "State_Machine_Class in"=w487) -> ("error out"=w484:errorcluster, "Elapsed Time(s)"=w482:dbl, "State_Machine_Class out"=w485:refnum<class "DIO.lvclass">)  [unwired: 6 in]
        n127 = Less Or Equal To 0?(x=w482) -> (x <= 0?=w483:bool)
        n128 = case shown="True" w483 {
          frame False {
          }
          frame True {
            n129 = local read "Lamp"() -> (w490:bool)
            n130 = Not(x=w490) -> (.not. x?=w489:bool)
            n131 = local write "Lamp"(w489) -> ()
          }
        }
      }
      frame "Messege_Confirm" {
        n132 = Variant To Data(error in=w493, type="", Variant=w496) -> (data=w491:string, error out=w492:errorcluster)
        n133 = One Button Dialog(message=w491) -> ()  [unwired: 1 in, 1 out]
      }
      frame "Set_Wait" {
        n134 = call-dynamic "State_Lock_Unlock.vi"("error in (no error)"=w500, "Parameter"=T4 {"Action_Mode (Get)"=enum."Set", "Action_Set (False)"=TRUE, "State_In (Wait)"="Wait"}, "State_Machine_Class in"=w501) -> ("error out"=w498:errorcluster, "State_Machine_Class out"=w499:refnum<class "DIO.lvclass">)  [unwired: 6 in, 1 out]
      }
      frame "Wait" {
        n135 = call-dynamic "State_Lock_Unlock.vi"("error in (no error)"=w505, "Parameter"=T4 {"Action_Mode (Get)"=enum."Get", "Action_Set (False)"=FALSE, "State_In (Wait)"="Wait"}, "State_Machine_Class in"=w506) -> ("error out"=w503:errorcluster, "State_Machine_Class out"=w504:refnum<class "DIO.lvclass">)  [unwired: 6 in, 1 out]
      }
      frame "Error_Action" {
        n136 = Variant To Data(error in=w510, type=w510, Variant=w509) -> (data=w511:errorcluster, error out=w508:errorcluster)
        n137 = call <vilib>:"Simple Error Handler.vi"("error in (no error)"=w511) -> ()  [unwired: 4 in, 5 out]
      }
      frame "Stop" {
        n138 = call-dynamic "State_Release.vi"("error in (no error)"=w520, "State_Machine_Class in"=w521) -> ("error out"=w518:errorcluster, "State_Machine_Class out"=w519:refnum<class "DIO.lvclass">)  [unwired: 8 in]
        n139 = call-dynamic "State_Lock_Unlock.vi"("error in (no error)"=w518, "Parameter"=T4 {"Action_Mode (Get)"=enum."Set", "Action_Set (False)"=TRUE, "State_In (Wait)"="Wait"}, "State_Machine_Class in"=w519) -> ("error out"=w515:errorcluster, "State_Machine_Class out"=w517:refnum<class "DIO.lvclass">)  [unwired: 6 in, 1 out]
        n140 = property on="Action Manager" class="Enum (strict)"(error in=w515, "Blinking"=TRUE) -> (error out=w514:errorcluster)  [unwired: 1 in, 1 out]
        n141 = One Button Dialog(message="All State is Locking !\nPlease Unlock With Action Manager to Release . . .") -> ()  [unwired: 1 in, 1 out]
      }
      frame "Exit" {
        n142 = call-dynamic "State_Release.vi"("error in (no error)"=w524, "State_Machine_Class in"=w525) -> ("error out"=w522:errorcluster, "State_Machine_Class out"=w523:refnum<class "DIO.lvclass">)  [unwired: 8 in]
      }
    }
    n143 = case shown="\"Init\"" w125 {
      tunnel: w147 -> [_ _ _ _ _ _ _ _ w390 _ _ w403 _ _]
      tunnel: w146 -> [w338 w340 w348 w350 w355 w364 w377 w384 w388 w395 w400 w402 w412 w416]
      tunnel: w145 -> [w337 w339 w347 w349 w354 w363 w376 w383 w387 w394 w399 w404 w411 w415]
      tunnel: [w335 w340 w344 w350 w353 w360 w375 w382 w388 w393 w398 w402 w407 w414] -> w140
      tunnel: [w334 w339 w343 w349 w352 w359 w374 w381 w386 w392 w397 w401 w406 w413] -> w139
      tunnel: w91 -> [w336 _ _ _ _ _ _ _ _ _ _ _ _ _]
      frame "Idle", Default {
        n144 = call-dynamic "State_Verify.vi"("error in (no error)"=w337, "State(Idle)"=w336, "State_Machine_Class in"=w338) -> ("error out"=w334:errorcluster, "Active"=→"Data_Logging":bool, "State_Machine_Class out"=w335:refnum<class "Data_Logging.lvclass">)  [unwired: 6 in]
      }
      frame "State_Interval" {
        # "Files Monitering or Cirtical Task Handling Here"
      }
      frame "Init" {
        n145 = call-dynamic "State_Interval.vi"("error in (no error)"=w347, "Parameter"=T5 {"Delay(s)"=15.0, "State (Interval_Delay)"="Interval_Delay"}, "State_Machine_Class in"=w348) -> ("error out"=w342:errorcluster, "State_Machine_Class out"=w345:refnum<class "Data_Logging.lvclass">)  [unwired: 6 in, 1 out]
        n146 = call-dynamic "State_Lock_Unlock.vi"("error in (no error)"=w342, "Parameter"=T4 {"Action_Mode (Get)"=enum."Set", "Action_Set (False)"=TRUE, "State_In (Wait)"="Wait"}, "State_Machine_Class in"=w345) -> ("error out"=w343:errorcluster, "State_Machine_Class out"=w344:refnum<class "Data_Logging.lvclass">)  [unwired: 6 in, 1 out]
      }
      frame "Data_Logging" {
        # "Save Data Files Here"
      }
      frame "Set_Interval" {
        n147 = call-dynamic "State_Interval.vi"("error in (no error)"=w354, "Parameter"=T5 {"Delay(s)"=15.0, "State (Interval_Delay)"="Interval_Delay"}, "State_Machine_Class in"=w355) -> ("error out"=w352:errorcluster, "State_Machine_Class out"=w353:refnum<class "Data_Logging.lvclass">)  [unwired: 6 in, 1 out]
      }
      frame "Interval_Delay" {
        n148 = call-dynamic "State_Interval.vi"("error in (no error)"=w363, "Parameter"=T5 {"Delay(s)"=0.0, "State (Interval_Delay)"="Interval_Delay"}, "State_Machine_Class in"=w364) -> ("error out"=w361:errorcluster, "Elapsed Time(s)"=w358:dbl, "State_Machine_Class out"=w362:refnum<class "Data_Logging.lvclass">)  [unwired: 6 in]
        n149 = local write "Data_Logging_Elapsed Time(s)"(w358) -> ()
        n150 = Less Or Equal To 0?(x=w358) -> (x <= 0?=w357:bool)
        n151 = local write "Data_Logging_Time_Act"(w357) -> ()
        n152 = case shown="True" w357 {
          tunnel: w362 -> [w366 w372]
          tunnel: w361 -> [w365 w371]
          tunnel: [w366 w370] -> w360
          tunnel: [w365 w369] -> w359
          frame False {
          }
          frame True {
            n153 = call-dynamic "State_LIFO.vi"("error in (no error)"=w371, "State_Interval(Enable)"=FALSE, "State Machine"=T2 {"Command"="Set_Interval", "Data"=variant} ("State"), "State_Machine_Class in"=w372) -> ("error out"=w369:errorcluster, "State_Machine_Class out"=w370:refnum<class "Data_Logging.lvclass">)  [unwired: 6 in]
          }
        }
      }
      frame "Set_Time_Out" {
        n154 = call-dynamic "State_Time_Out.vi"("error in (no error)"=w376, "Parameter"=T3 {"Enable(True)"=TRUE, "Time Out_State Name"="Get_Time_Out", "Time Target (1s)"=30.0, "Time Out_Reply Message_State"="Interval_Delay"}, "State_Machine_Class in"=w377) -> ("error out"=w374:errorcluster, "State_Machine_Class out"=w375:refnum<class "Data_Logging.lvclass">)  [unwired: 5 in, 2 out]
      }
      frame "Get_Time_Out" {
        # "Messege_Confirm"
        n155 = call-dynamic "State_Time_Out.vi"("error in (no error)"=w383, "Parameter"=T3 {"Enable(True)"=TRUE, "Time Out_State Name"="Get_Time_Out", "Time Target (1s)"=0.0, "Time Out_Reply Message_State"="Messege_Confirm"}, "State_Machine_Class in"=w384) -> ("error out"=w381:errorcluster, "Remaining Time (s)"=→"Data_Logging_Elapsed Time(s)":dbl, "Timeout"=→"Data_Logging_Time_Act":bool, "State_Machine_Class out"=w382:refnum<class "Data_Logging.lvclass">)  [unwired: 5 in]
      }
      frame "Messege_Confirm" {
        n156 = Variant To Data(error in=w387, type="", Variant=w390) -> (data=w385:string, error out=w386:errorcluster)
        n157 = One Button Dialog(message=w385) -> ()  [unwired: 1 in, 1 out]
      }
      frame "Set_Wait" {
        n158 = call-dynamic "State_Lock_Unlock.vi"("error in (no error)"=w394, "Parameter"=T4 {"Action_Mode (Get)"=enum."Set", "Action_Set (False)"=TRUE, "State_In (Wait)"="Wait"}, "State_Machine_Class in"=w395) -> ("error out"=w392:errorcluster, "State_Machine_Class out"=w393:refnum<class "Data_Logging.lvclass">)  [unwired: 6 in, 1 out]
      }
      frame "Wait" {
        n159 = call-dynamic "State_Lock_Unlock.vi"("error in (no error)"=w399, "Parameter"=T4 {"Action_Mode (Get)"=enum."Get", "Action_Set (False)"=TRUE, "State_In (Wait)"="Wait"}, "State_Machine_Class in"=w400) -> ("error out"=w397:errorcluster, "State_Machine_Class out"=w398:refnum<class "Data_Logging.lvclass">)  [unwired: 6 in, 1 out]
      }
      frame "Error_Action" {
        n160 = Variant To Data(error in=w404, type=w404, Variant=w403) -> (data=w405:errorcluster, error out=w401:errorcluster)
        n161 = call <vilib>:"Simple Error Handler.vi"("error in (no error)"=w405) -> ()  [unwired: 4 in, 5 out]
      }
      frame "Stop" {
        n162 = call-dynamic "State_Release.vi"("error in (no error)"=w411, "State_Machine_Class in"=w412) -> ("error out"=w409:errorcluster, "State_Machine_Class out"=w410:refnum<class "Data_Logging.lvclass">)  [unwired: 8 in]
        n163 = call-dynamic "State_Lock_Unlock.vi"("error in (no error)"=w409, "Parameter"=T4 {"Action_Mode (Get)"=enum."Set", "Action_Set (False)"=TRUE, "State_In (Wait)"="Wait"}, "State_Machine_Class in"=w410) -> ("error out"=w406:errorcluster, "State_Machine_Class out"=w407:refnum<class "Data_Logging.lvclass">)  [unwired: 6 in, 1 out]
      }
      frame "Exit" {
        n164 = call-dynamic "State_Release.vi"("error in (no error)"=w415, "State_Machine_Class in"=w416) -> ("error out"=w413:errorcluster, "State_Machine_Class out"=w414:refnum<class "Data_Logging.lvclass">)  [unwired: 8 in]
      }
    }
    n165 = case shown="\"Init\"" w104 {
      tunnel: w109 -> [_ _ _ _ _ _ _ w306 _ _ w320 _ _]
      tunnel: w75 -> [w256 w258 w266 w271 w272 w293 w300 w304 w311 w316 w318 w328 w332]
      tunnel: w110 -> [w255 w257 w265 w270 w280 w292 w299 w303 w310 w315 w319 w327 w331]
      tunnel: [w253 w258 w260 w269 w277 w291 w298 w304 w309 w314 w318 w323 w330] -> w111
      tunnel: [w252 w257 w259 w268 w276 w290 w297 w302 w308 w313 w317 w322 w329] -> w112
      tunnel: w90 -> [w254 _ _ _ _ _ _ _ _ _ _ _ _]
      frame "Idle", Default {
        n166 = call-dynamic "State_Verify.vi"("error in (no error)"=w255, "State(Idle)"=w254, "State_Machine_Class in"=w256) -> ("error out"=w252:errorcluster, "Active"=→"Common":bool, "State_Machine_Class out"=w253:refnum<class "Common_State.lvclass">)  [unwired: 6 in]
      }
      frame "State_Interval" {
        # "Cirtical Task Handling Here"
      }
      frame "Init" {
        n167 = call-dynamic "State_Interval.vi"("error in (no error)"=w265, "Parameter"=T5 {"Delay(s)"=15.0, "State (Interval_Delay)"="Interval_Delay"}, "State_Machine_Class in"=w266) -> ("error out"=w262:errorcluster, "State_Machine_Class out"=w263:refnum<class "Common_State.lvclass">)  [unwired: 6 in, 1 out]
        n168 = call-dynamic "State_Lock_Unlock.vi"("error in (no error)"=w262, "Parameter"=T4 {"Action_Mode (Get)"=enum."Set", "Action_Set (False)"=TRUE, "State_In (Wait)"="Wait"}, "State_Machine_Class in"=w263) -> ("error out"=w259:errorcluster, "State_Machine_Class out"=w260:refnum<class "Common_State.lvclass">)  [unwired: 6 in, 1 out]
      }
      frame "Set_Interval" {
        n169 = call-dynamic "State_Interval.vi"("error in (no error)"=w270, "Parameter"=T5 {"Delay(s)"=15.0, "State (Interval_Delay)"="Interval_Delay"}, "State_Machine_Class in"=w271) -> ("error out"=w268:errorcluster, "State_Machine_Class out"=w269:refnum<class "Common_State.lvclass">)  [unwired: 6 in, 1 out]
      }
      frame "Interval_Delay" {
        n170 = call-dynamic "State_Interval.vi"("error in (no error)"=w280, "Parameter"=T5 {"Delay(s)"=5.0, "State (Interval_Delay)"="Interval_Delay"}, "State_Machine_Class in"=w272) -> ("error out"=w278:errorcluster, "Elapsed Time(s)"=w275:dbl, "State_Machine_Class out"=w279:refnum<class "Common_State.lvclass">)  [unwired: 6 in]
        n171 = local write "Common_Elapsed Time(s)"(w275) -> ()
        n172 = Less Or Equal To 0?(x=w275) -> (x <= 0?=w274:bool)
        n173 = local write "Common_Time_Act"(w274) -> ()
        n174 = case shown="True" w274 {
          tunnel: w279 -> [w282 w288]
          tunnel: w278 -> [w281 w287]
          tunnel: [w282 w286] -> w277
          tunnel: [w281 w285] -> w276
          frame False {
          }
          frame True {
            n175 = call-dynamic "State_LIFO.vi"("error in (no error)"=w287, "State_Interval(Enable)"=FALSE, "State Machine"=T2 {"Command"="Interval_Delay", "Data"=variant} ("State"), "State_Machine_Class in"=w288) -> ("error out"=w285:errorcluster, "State_Machine_Class out"=w286:refnum<class "Common_State.lvclass">)  [unwired: 6 in]
          }
        }
      }
      frame "Set_Time_Out" {
        n176 = call-dynamic "State_Time_Out.vi"("error in (no error)"=w292, "Parameter"=T3 {"Enable(True)"=TRUE, "Time Out_State Name"="Get_Time_Out", "Time Target (1s)"=30.0, "Time Out_Reply Message_State"="Interval_Delay"}, "State_Machine_Class in"=w293) -> ("error out"=w290:errorcluster, "State_Machine_Class out"=w291:refnum<class "Common_State.lvclass">)  [unwired: 5 in, 2 out]
      }
      frame "Get_Time_Out" {
        # "Messege_Confirm"
        # "Messege_Confirm"
        n177 = call-dynamic "State_Time_Out.vi"("error in (no error)"=w299, "Parameter"=T3 {"Enable(True)"=TRUE, "Time Out_State Name"="Get_Time_Out", "Time Target (1s)"=0.0, "Time Out_Reply Message_State"="Set_Interval"}, "State_Machine_Class in"=w300) -> ("error out"=w297:errorcluster, "Remaining Time (s)"=→"Common_Elapsed Time(s)":dbl, "Timeout"=→"Common_Time_Act":bool, "State_Machine_Class out"=w298:refnum<class "Common_State.lvclass">)  [unwired: 5 in]
      }
      frame "Messege_Confirm" {
        n178 = Variant To Data(error in=w303, type="", Variant=w306) -> (data=w301:string, error out=w302:errorcluster)
        n179 = One Button Dialog(message=w301) -> ()  [unwired: 1 in, 1 out]
      }
      frame "Set_Wait" {
        n180 = call-dynamic "State_Lock_Unlock.vi"("error in (no error)"=w310, "Parameter"=T4 {"Action_Mode (Get)"=enum."Set", "Action_Set (False)"=TRUE, "State_In (Wait)"="Wait"}, "State_Machine_Class in"=w311) -> ("error out"=w308:errorcluster, "State_Machine_Class out"=w309:refnum<class "Common_State.lvclass">)  [unwired: 6 in, 1 out]
      }
      frame "Wait" {
        n181 = call-dynamic "State_Lock_Unlock.vi"("error in (no error)"=w315, "Parameter"=T4 {"Action_Mode (Get)"=enum."Get", "Action_Set (False)"=FALSE, "State_In (Wait)"="Wait"}, "State_Machine_Class in"=w316) -> ("error out"=w313:errorcluster, "State_Machine_Class out"=w314:refnum<class "Common_State.lvclass">)  [unwired: 6 in, 1 out]
      }
      frame "Error_Action" {
        n182 = Variant To Data(error in=w319, type=w319, Variant=w320) -> (data=w321:errorcluster, error out=w317:errorcluster)
        n183 = call <vilib>:"Simple Error Handler.vi"("error in (no error)"=w321) -> ()  [unwired: 4 in, 5 out]
      }
      frame "Stop" {
        n184 = call-dynamic "State_Release.vi"("error in (no error)"=w327, "State_Machine_Class in"=w328) -> ("error out"=w325:errorcluster, "State_Machine_Class out"=w326:refnum<class "Common_State.lvclass">)  [unwired: 8 in]
        n185 = call-dynamic "State_Lock_Unlock.vi"("error in (no error)"=w325, "Parameter"=T4 {"Action_Mode (Get)"=enum."Set", "Action_Set (False)"=TRUE, "State_In (Wait)"="Wait"}, "State_Machine_Class in"=w326) -> ("error out"=w322:errorcluster, "State_Machine_Class out"=w323:refnum<class "Common_State.lvclass">)  [unwired: 6 in, 1 out]
      }
      frame "Exit" {
        n186 = call-dynamic "State_Release.vi"("error in (no error)"=w331, "State_Machine_Class in"=w332) -> ("error out"=w329:errorcluster, "State_Machine_Class out"=w330:refnum<class "Common_State.lvclass">)  [unwired: 8 in]
      }
    }
    n187 = case shown="\"Init\"" w87 {
      tunnel: w84 -> [_ _ _ _ _ _ _ w224 _ _ w238 _ _]
      tunnel: w83 -> [w175 w177 w181 w190 w199 w211 w218 w222 w229 w234 w236 w246 w250]
      tunnel: w82 -> [w174 w176 w179 w189 w198 w210 w217 w221 w228 w233 w237 w245 w249]
      tunnel: [w172 w177 w185 w188 w195 w209 w216 w222 w227 w232 w236 w241 w248] -> w80
      tunnel: [w171 w176 w184 w187 w194 w208 w215 w220 w226 w231 w235 w240 w247] -> w78
      tunnel: w79 -> [w173 _ _ _ _ _ _ _ _ _ _ _ _]
      frame "Idle", Default {
        n188 = call-dynamic "State_Verify.vi"("error in (no error)"=w174, "State(Idle)"=w173, "State_Machine_Class in"=w175) -> ("error out"=w171:errorcluster, "Active"=→"Base Class":bool, "State_Machine_Class out"=w172:refnum<class "Hyper_State_Machine.lvclass">)  [unwired: 6 in]
      }
      frame "State_Interval" {
        # "Cirtical Task Handling Here"
      }
      frame "Init" {
        n189 = call-dynamic "State_Time_Out.vi"("error in (no error)"=w179, "Parameter"=T3 {"Enable(True)"=TRUE, "Time Out_State Name"="Get_Time_Out", "Time Target (1s)"=10.0, "Time Out_Reply Message_State"="Get_Time_Out"}, "State_Machine_Class in"=w181) -> ("error out"=w178:errorcluster, "State_Machine_Class out"=w180:refnum<class "Hyper_State_Machine.lvclass">)  [unwired: 5 in, 2 out]
        n190 = call-dynamic "State_Lock_Unlock.vi"("error in (no error)"=w178, "Parameter"=T4 {"Action_Mode (Get)"=enum."Set", "Action_Set (False)"=TRUE, "State_In (Wait)"="Wait"}, "State_Machine_Class in"=w180) -> ("error out"=w184:errorcluster, "State_Machine_Class out"=w185:refnum<class "Hyper_State_Machine.lvclass">)  [unwired: 6 in, 1 out]
      }
      frame "Set_Interval" {
        n191 = call-dynamic "State_Interval.vi"("error in (no error)"=w189, "Parameter"=T5 {"Delay(s)"=15.0, "State (Interval_Delay)"="Interval_Delay"}, "State_Machine_Class in"=w190) -> ("error out"=w187:errorcluster, "State_Machine_Class out"=w188:refnum<class "Hyper_State_Machine.lvclass">)  [unwired: 6 in, 1 out]
      }
      frame "Interval_Delay" {
        n192 = call-dynamic "State_Interval.vi"("error in (no error)"=w198, "Parameter"=T5 {"Delay(s)"=0.0, "State (Interval_Delay)"="Interval_Delay"}, "State_Machine_Class in"=w199) -> ("error out"=w196:errorcluster, "Elapsed Time(s)"=w193:dbl, "State_Machine_Class out"=w197:refnum<class "Hyper_State_Machine.lvclass">)  [unwired: 6 in]
        n193 = local write "Base Class_Elapsed Time(s)"(w193) -> ()
        n194 = Less Or Equal To 0?(x=w193) -> (x <= 0?=w192:bool)
        n195 = local write "Base Class_Time_Act"(w192) -> ()
        n196 = case shown="True" w192 {
          tunnel: w197 -> [w201 w206]
          tunnel: w196 -> [w200 w205]
          tunnel: [w201 w204] -> w195
          tunnel: [w200 w203] -> w194
          frame False {
          }
          frame True {
            n197 = call-dynamic "State_LIFO.vi"("error in (no error)"=w205, "State Machine"=T2 {"Command"="Set_Interval", "Data"=variant} ("State"), "State_Machine_Class in"=w206) -> ("error out"=w203:errorcluster, "State_Machine_Class out"=w204:refnum<class "Hyper_State_Machine.lvclass">)  [unwired: 7 in]
          }
        }
      }
      frame "Set_Time_Out" {
        n198 = call-dynamic "State_Time_Out.vi"("error in (no error)"=w210, "Parameter"=T3 {"Enable(True)"=TRUE, "Time Out_State Name"="Get_Time_Out", "Time Target (1s)"=30.0, "Time Out_Reply Message_State"="Interval_Delay"}, "State_Machine_Class in"=w211) -> ("error out"=w208:errorcluster, "State_Machine_Class out"=w209:refnum<class "Hyper_State_Machine.lvclass">)  [unwired: 5 in, 2 out]
      }
      frame "Get_Time_Out" {
        # "Messege_Confirm"
        n199 = call-dynamic "State_Time_Out.vi"("error in (no error)"=w217, "Parameter"=T3 {"Enable(True)"=TRUE, "Time Out_State Name"="Get_Time_Out", "Time Target (1s)"=5.0, "Time Out_Reply Message_State"="Get_Time_Out"}, "State_Machine_Class in"=w218) -> ("error out"=w215:errorcluster, "Remaining Time (s)"=→"Base Class_Elapsed Time(s)":dbl, "Timeout"=→"Base Class_Time_Act":bool, "State_Machine_Class out"=w216:refnum<class "Hyper_State_Machine.lvclass">)  [unwired: 5 in]
      }
      frame "Messege_Confirm" {
        n200 = Variant To Data(error in=w221, type="", Variant=w224) -> (data=w219:string, error out=w220:errorcluster)
        n201 = One Button Dialog(message=w219) -> ()  [unwired: 1 in, 1 out]
      }
      frame "Set_Wait" {
        n202 = call-dynamic "State_Lock_Unlock.vi"("error in (no error)"=w228, "Parameter"=T4 {"Action_Mode (Get)"=enum."Set", "Action_Set (False)"=TRUE, "State_In (Wait)"="Wait"}, "State_Machine_Class in"=w229) -> ("error out"=w226:errorcluster, "State_Machine_Class out"=w227:refnum<class "Hyper_State_Machine.lvclass">)  [unwired: 6 in, 1 out]
      }
      frame "Wait" {
        n203 = call-dynamic "State_Lock_Unlock.vi"("error in (no error)"=w233, "Parameter"=T4 {"Action_Mode (Get)"=enum."Get", "Action_Set (False)"=FALSE, "State_In (Wait)"="Wait"}, "State_Machine_Class in"=w234) -> ("error out"=w231:errorcluster, "State_Machine_Class out"=w232:refnum<class "Hyper_State_Machine.lvclass">)  [unwired: 6 in, 1 out]
      }
      frame "Error_Action" {
        n204 = Variant To Data(error in=w237, type=w237, Variant=w238) -> (data=w239:errorcluster, error out=w235:errorcluster)
        n205 = call <vilib>:"Simple Error Handler.vi"("error in (no error)"=w239) -> ()  [unwired: 4 in, 5 out]
      }
      frame "Stop" {
        n206 = call-dynamic "State_Release.vi"("error in (no error)"=w245, "State_Machine_Class in"=w246) -> ("error out"=w243:errorcluster, "State_Machine_Class out"=w244:refnum<class "Hyper_State_Machine.lvclass">)  [unwired: 8 in]
        n207 = call-dynamic "State_Lock_Unlock.vi"("error in (no error)"=w243, "Parameter"=T4 {"Action_Mode (Get)"=enum."Set", "Action_Set (False)"=TRUE, "State_In (Wait)"="Wait"}, "State_Machine_Class in"=w244) -> ("error out"=w240:errorcluster, "State_Machine_Class out"=w241:refnum<class "Hyper_State_Machine.lvclass">)  [unwired: 6 in, 1 out]
      }
      frame "Exit" {
        n208 = call-dynamic "State_Release.vi"("error in (no error)"=w249, "State_Machine_Class in"=w250) -> ("error out"=w247:errorcluster, "State_Machine_Class out"=w248:refnum<class "Hyper_State_Machine.lvclass">)  [unwired: 8 in]
      }
    }
    n209 = case "Commander" shown="\"Init\"" w169 {
      tunnel: w168 -> [_ _ _ _ _ _ _ w821 w829 _ _ _ w857 _ _]
      tunnel: w166 -> [w756 w758 w765 w783 w793 w808 w815 w819 w825 w834 w849 w853 w858 w865 w870]
      tunnel: w165 -> [w754 w757 w764 w782 w792 w807 w814 w818 w828 w833 w848 w852 w854 w864 w869]
      tunnel: [w753 w758 w767 w781 w788 w806 w813 w819 w825 w832 w847 w851 w858 w861 w868] -> w96
      tunnel: [w752 w757 w766 w780 w787 w805 w812 w817 w824 w837 w846 w850 w855 w860 w867] -> w164
      tunnel: [_ _ _ _ _ _ _ _ _ _ _ _ _ _ TRUE] -> w167
      tunnel: w95 -> [w755 _ _ _ w784 _ _ _ _ _ _ _ _ _ _]
      frame "Idle", Default {
        n210 = call-dynamic "State_Verify.vi"("error in (no error)"=w754, "State(Idle)"=w755, "State_Machine_Class in"=w756) -> ("error out"=w752:errorcluster, "Active"=→"Commander":bool, "State_Machine_Class out"=w753:refnum<class "Commander.lvclass">)  [unwired: 6 in]
      }
      frame "State_Interval" {
      }
      frame "Init" {
        # "Test Using Static Delay (2s) + SetInterval (3s) = 5 sec"
        n211 = call-dynamic "Product_Activate.vi"("error in (no error)"=w764, "Activate Code"="Activate_Code(Blank for 30 min Trial)", "Commander in"=w765) -> ("error out"=w762:errorcluster, "Activate"=→"Activate":bool, "Product ID"=→"Product ID":string, "Commander out"=w763:refnum<class "Commander.lvclass">)  [unwired: 5 in]
        n212 = disable-structure shown="Enabled" {
          disable-tunnel: [w772 w777] -> w767
          disable-tunnel: [w771 w776] -> w766
          disable-tunnel: w763 -> [w769 w778]
          disable-tunnel: w762 -> [w768 w775]
          frame Disabled {
            n213 = call-dynamic "State_Interval.vi"("error in (no error)"=w768, "Parameter"=T5 {"Delay(s)"=5.0, "State (Interval_Delay)"="Interval_Delay"}, "State_Machine_Class in"=w769) -> ("error out"=w771:errorcluster, "State_Machine_Class out"=w772:refnum<class "Commander.lvclass">)  [unwired: 6 in, 1 out]
          }
          frame Enabled {
            n214 = Build Array(T2 {"Command"="Interval_Delay", "Data"=variant} ("State")) -> (w773:T2[])
            n215 = call-dynamic "State_FIFO.vi"("error in (no error)"=w775, "State Machine[]"=w773, "State_Machine_Class in"=w778) -> ("error out"=w776:errorcluster, "State_Machine_Class out"=w777:refnum<class "Commander.lvclass">)  [unwired: 7 in]
          }
        }
      }
      frame "Set_Interval" {
        n216 = call-dynamic "State_Interval.vi"("error in (no error)"=w782, "Parameter"=T5 {"Delay(s)"=3.0, "State (Interval_Delay)"="Interval_Delay"}, "State_Machine_Class in"=w783) -> ("error out"=w780:errorcluster, "State_Machine_Class out"=w781:refnum<class "Commander.lvclass">)  [unwired: 6 in, 1 out]
      }
      frame "Interval_Delay" {
        n217 = call-dynamic "State_Interval.vi"("error in (no error)"=w792, "Parameter"=T5 {"Delay(s)"=5.0, "State (Interval_Delay)"="Interval_Delay"}, "State_Machine_Class in"=w793) -> ("error out"=w789:errorcluster, "Elapsed Time(s)"=w786:dbl, "State_Machine_Class out"=w790:refnum<class "Commander.lvclass">)  [unwired: 6 in]
        "Commander_Elapsed Time(s)" <- w786
        n218 = Less Or Equal To 0?(x=w786) -> (x <= 0?=w791:bool)
        n219 = local write "State1_Time_Act"(w791) -> ()
        n220 = case shown="True" w791 {
          tunnel: w790 -> [w795 w803]
          tunnel: w789 -> [w794 w802]
          tunnel: [w795 w801] -> w788
          tunnel: [w794 w800] -> w787
          tunnel: w784 -> [_ w796]
          frame False {
          }
          frame True {
            n221 = Build Array(T2 {"Command"="Member_Release", "Data"=variant} ("State"), T2 {"Command"="Set_Interval", "Data"=variant} ("State"), w796) -> (w799:T2[])
            n222 = call-dynamic "State_FIFO.vi"("error in (no error)"=w802, "State Machine[]"=w799, "State_Machine_Class in"=w803) -> ("error out"=w800:errorcluster, "State_Machine_Class out"=w801:refnum<class "Commander.lvclass">)  [unwired: 7 in]
          }
        }
      }
      frame "Set_Time_Out" {
        n223 = call-dynamic "State_Time_Out.vi"("error in (no error)"=w807, "Parameter"=T3 {"Enable(True)"=TRUE, "Time Out_State Name"="Get_Time_Out", "Time Target (1s)"=30.0, "Time Out_Reply Message_State"="Messege_Confirm"}, "State_Machine_Class in"=w808) -> ("error out"=w805:errorcluster, "State_Machine_Class out"=w806:refnum<class "Commander.lvclass">)  [unwired: 5 in, 2 out]
      }
      frame "Get_Time_Out" {
        n224 = call-dynamic "State_Time_Out.vi"("error in (no error)"=w814, "Parameter"=T3 {"Enable(True)"=TRUE, "Time Out_State Name"="Get_Time_Out", "Time Target (1s)"=0.0, "Time Out_Reply Message_State"="Messege_Confirm"}, "State_Machine_Class in"=w815) -> ("error out"=w812:errorcluster, "Remaining Time (s)"=w811:dbl, "Timeout"=→"State1_Time_Act":bool, "State_Machine_Class out"=w813:refnum<class "Commander.lvclass">)  [unwired: 5 in]
        n225 = local write "Commander_Elapsed Time(s)"(w811) -> ()
      }
      frame "Messege_Confirm" {
        n226 = Variant To Data(error in=w818, type="", Variant=w821) -> (data=w816:string, error out=w817:errorcluster)
        n227 = One Button Dialog(message=w816) -> ()  [unwired: 1 in, 1 out]
      }
      frame "Dynamics_Release" {
        n228 = Variant To Data(error in=w828, type=refnum<class "Hyper_State_Machine.lvclass"> refnum ("SSW_Hyper_State_Machine.lvlibp:Hyper_State_Machine.lvclass"), Variant=w829) -> (data=w827:refnum<class "Hyper_State_Machine.lvclass">, error out=w826:errorcluster)
        n229 = call-dynamic "State_Lock_Unlock.vi"("error in (no error)"=w826, "Parameter"=T4 {"Action_Mode (Get)"=enum."Set", "Action_Set (False)"=FALSE, "State_In (Wait)"="Wait"}, "State_Machine_Class in"=w827) -> ("error out"=w824:errorcluster)  [unwired: 6 in, 2 out]
      }
      frame "Member_Release" {
        (unwired) refnum<class "Commander.lvclass"> refnum ("Commander.lvclass")
        # "This method the CMD Class is do not yet to override Parent Class so using Parent Method"
        n230 = call-dynamic "Get_Child_State.vi"("error in (no error)"=w833, "Hyper_State_Machine in"=w834) -> ("error out"=w830:errorcluster, "Child_State"=w831:refnum<class "State_Interface.lvclass">[], "Hyper_State_Machine out"=w832:refnum<class "Commander.lvclass">)  [unwired: 5 in, 2 out]
        n231 = for {
          tunnel: w831 -> [w843] mode=indexing
          shift-right: [w844] -> w837
          shift-left: w830 -> [w841]
          tunnel: refnum<class "Hyper_State_Machine.lvclass"> refnum ("SSW_Hyper_State_Machine.lvlibp:Hyper_State_Machine.lvclass") -> [w839]
          tunnel: T4 {"Action_Mode (Get)"=enum."Set", "Action_Set (False)"=FALSE, "State_In (Wait)"="Wait"} ("Parameter") -> [w838]
          n232 = To More Specific Class(target class=w839, reference=w843, error in=w841) -> (specific class reference=w842:refnum<class "Hyper_State_Machine.lvclass">, error out=w840:errorcluster)
          n233 = call-dynamic "State_Lock_Unlock.vi"("error in (no error)"=w840, "Parameter"=w838, "State_Machine_Class in"=w842) -> ("error out"=w844:errorcluster)  [unwired: 6 in, 2 out]
        }
      }
      frame "Set_Wait" {
        n234 = call-dynamic "State_Lock_Unlock.vi"("error in (no error)"=w848, "Parameter"=T4 {"Action_Mode (Get)"=enum."Set", "Action_Set (False)"=TRUE, "State_In (Wait)"="Wait"}, "State_Machine_Class in"=w849) -> ("error out"=w846:errorcluster, "State_Machine_Class out"=w847:refnum<class "Commander.lvclass">)  [unwired: 6 in, 1 out]
      }
      frame "Wait" {
        n235 = call-dynamic "State_Lock_Unlock.vi"("error in (no error)"=w852, "State_Machine_Class in"=w853) -> ("error out"=w850:errorcluster, "State_Machine_Class out"=w851:refnum<class "Commander.lvclass">)  [unwired: 7 in, 1 out]
      }
      frame "Error_Action" {
        n236 = Variant To Data(error in=w854, type=w854, Variant=w857) -> (data=w856:errorcluster, error out=w855:errorcluster)
        n237 = call <vilib>:"Simple Error Handler.vi"("error in (no error)"=w856) -> ()  [unwired: 4 in, 5 out]
      }
      frame "Stop" {
        n238 = call-dynamic "State_Release.vi"("error in (no error)"=w864, "State_Machine_Class in"=w865) -> ("error out"=w862:errorcluster, "State_Machine_Class out"=w863:refnum<class "Commander.lvclass">)  [unwired: 8 in]
        n239 = call-dynamic "State_Lock_Unlock.vi"("error in (no error)"=w862, "Parameter"=T4 {"Action_Mode (Get)"=enum."Set", "Action_Set (False)"=TRUE, "State_In (Wait)"="Wait"}, "State_Machine_Class in"=w863) -> ("error out"=w860:errorcluster, "State_Machine_Class out"=w861:refnum<class "Commander.lvclass">)  [unwired: 6 in, 1 out]
      }
      frame "Exit" {
        n240 = call-dynamic "State_Release.vi"("error in (no error)"=w869, "State_Machine_Class in"=w870) -> ("error out"=w867:errorcluster, "State_Machine_Class out"=w868:refnum<class "Commander.lvclass">)  [unwired: 8 in]
      }
    }
    n241 = local read "Heart_Rate"() -> (w73:bool)
    n242 = Or(x=w167, y=w154) -> (x .or. y?=w155:bool)
    n243 = Not(x=w73) -> (.not. x?=→"Heart_Rate":bool)
    n244 = call <vilib>:"High Resolution Polling Wait.vi"("seconds to wait"="System_Wait_Time") -> ()  [unwired: 10 in, 1 out]
    n245 = call-dynamic "State_Error_Handling.vi"("error in (no error)"=w150, "Reply_State_Name"=w76, "Handling_State(State_Acquisition)"=w94, "State_Machine_Class in"=w151) -> ("error out"=w157:errorcluster)  [unwired: 6 in, 1 out]
    n246 = call-dynamic "State_Error_Handling.vi"("error in (no error)"=w135, "Reply_State_Name"=w76, "Handling_State(State_Acquisition)"=w93, "State_Machine_Class in"=w138) -> ("error out"=w131:errorcluster)  [unwired: 6 in, 1 out]
    n247 = call-dynamic "State_Error_Handling.vi"("error in (no error)"=w141, "Reply_State_Name"=w76, "Handling_State(State_Acquisition)"=w92, "State_Machine_Class in"=w142) -> ("error out"=w130:errorcluster)  [unwired: 6 in, 1 out]
    n248 = call-dynamic "State_Error_Handling.vi"("error in (no error)"=w139, "Reply_State_Name"=w76, "Handling_State(State_Acquisition)"=w91, "State_Machine_Class in"=w140) -> ("error out"=w129:errorcluster)  [unwired: 6 in, 1 out]
    n249 = call-dynamic "State_Error_Handling.vi"("error in (no error)"=w112, "Reply_State_Name"=w76, "Handling_State(State_Acquisition)"=w90, "State_Machine_Class in"=w111) -> ("error out"=w107:errorcluster)  [unwired: 6 in, 1 out]
    n250 = call-dynamic "State_Error_Handling.vi"("error in (no error)"=w78, "Reply_State_Name"=w76, "Handling_State(State_Acquisition)"=w79, "State_Machine_Class in"=w80) -> ("error out"=w77:errorcluster)  [unwired: 6 in, 1 out]
    n251 = call-dynamic "State_Error_Handling.vi"("error in (no error)"=w164, "Reply_State_Name"=w76, "Handling_State(State_Acquisition)"=w95, "State_Machine_Class in"=w96) -> ("error out"=w163:errorcluster, "State_Machine_Class out"=w162:refnum<class "Commander.lvclass">)  [unwired: 6 in]
  }
  n252 = while {
    tunnel: w16 -> [w871]
    stop <- w872 stop-if-true
    n253 = event shown="[2] \"Stop\": Value Change" {
      selector: _ -> [_ _ _]
      dyn-events: _ -> [_ _ _]
      timeout: _ -> [_ _ _]
      tunnel: [_ _ TRUE] -> w872
      tunnel: w871 -> [_ w877 w935]
      event Timeout {
        n254 = event-data() -> ()  [unwired: 1 in, 3 out]
      }
      event "Action Manager": Value Change {
        n255 = event-data() -> ("NewVal"=w882:T1)  [unwired: 1 in]
        n256 = call-dynamic "Get_Child_State.vi"("error in (no error)"=errorcluster {"status"=FALSE, "code"=0, "source"=""} ("error out"), "Hyper_State_Machine in"=w877) -> ("error out"=w873:errorcluster, "Child_State"=w874:refnum<class "State_Interface.lvclass">[], "Hyper_State_Machine out"=w875:refnum<class "Commander.lvclass">)  [unwired: 5 in, 2 out]
        n257 = Build Array (concatenate)(w875, w874) -> (w879:refnum<class "State_Interface.lvclass">[])
        n258 = case shown="\"Lock\"" w882 {
          tunnel: w879 -> [_ w888 w901 w913 w924]
          tunnel: [w883 w886 w900 w912 w922] -> w881
          tunnel: w873 -> [w883 w887 w899 w911 w923]
          tunnel: refnum<class "Hyper_State_Machine.lvclass"> refnum ("SSW_Hyper_State_Machine.lvlibp:Hyper_State_Machine.lvclass") -> [_ w884 w897 w909 w921]
          frame "No Action", Default {
          }
          frame "Init" {
            n259 = for {
              tunnel: w888 -> [w894] mode=indexing
              shift-right: [w895] -> w886
              shift-left: w887 -> [w890]
              tunnel: w884 -> [w892]
              tunnel: T2 {"Command"="Init", "Data"=variant} ("State") -> [w891]
              n260 = To More Specific Class(target class=w892, reference=w894, error in=w890) -> (specific class reference=w893:refnum<class "Hyper_State_Machine.lvclass">, error out=w889:errorcluster)
              n261 = call-dynamic "State_LIFO.vi"("error in (no error)"=w889, "State_Interval(Enable)"=FALSE, "State Machine"=w891, "State_Machine_Class in"=w893) -> ("error out"=w895:errorcluster)  [unwired: 6 in, 1 out]
            }
          }
          frame "Lock" {
            n262 = for {
              tunnel: w901 -> [w907] mode=indexing
              shift-right: [w908] -> w900
              shift-left: w899 -> [w903]
              tunnel: w897 -> [w906]
              tunnel: T4 {"Action_Mode (Get)"=enum."Set", "Action_Set (False)"=TRUE, "State_In (Wait)"="Wait"} ("Parameter") -> [w904]
              n263 = To More Specific Class(target class=w906, reference=w907, error in=w903) -> (specific class reference=w905:refnum<class "Hyper_State_Machine.lvclass">, error out=w902:errorcluster)
              n264 = call-dynamic "State_Lock_Unlock.vi"("error in (no error)"=w902, "Parameter"=w904, "State_Machine_Class in"=w905) -> ("error out"=w908:errorcluster)  [unwired: 6 in, 2 out]
            }
          }
          frame "Unlock" {
            n265 = for {
              tunnel: w913 -> [w918] mode=indexing
              shift-right: [w920] -> w912
              shift-left: w911 -> [w915]
              tunnel: T4 {"Action_Mode (Get)"=enum."Set", "Action_Set (False)"=FALSE, "State_In (Wait)"="Wait"} ("Parameter") -> [w919]
              tunnel: w909 -> [w917]
              n266 = To More Specific Class(target class=w917, reference=w918, error in=w915) -> (specific class reference=w916:refnum<class "Hyper_State_Machine.lvclass">, error out=w914:errorcluster)
              n267 = call-dynamic "State_Lock_Unlock.vi"("error in (no error)"=w914, "Parameter"=w919, "State_Machine_Class in"=w916) -> ("error out"=w920:errorcluster)  [unwired: 6 in, 2 out]
            }
          }
          frame "Release" {
            n268 = for {
              tunnel: w924 -> [w929] mode=indexing
              shift-right: [w930] -> w922
              shift-left: w923 -> [w926]
              tunnel: w921 -> [w928]
              n269 = To More Specific Class(target class=w928, reference=w929, error in=w926) -> (specific class reference=w927:refnum<class "Hyper_State_Machine.lvclass">, error out=w925:errorcluster)
              n270 = call-dynamic "State_Release.vi"("error in (no error)"=w925, "State_Machine_Class in"=w927) -> ("error out"=w930:errorcluster)  [unwired: 8 in, 1 out]
            }
          }
        }
        n271 = property on="Action Manager" class="Enum (strict)"(error in=w881, "Blinking"=FALSE) -> ()  [unwired: 1 in, 2 out]
      }
      event "Stop": Value Change {
        n272 = event-data() -> ()  [unwired: 1 in, 6 out]
        n273 = call-dynamic "Get_Child_State.vi"("error in (no error)"=errorcluster {"status"=FALSE, "code"=0, "source"=""} ("error out"), "Hyper_State_Machine in"=w935) -> ("error out"=w931:errorcluster, "Child_State"=w932:refnum<class "State_Interface.lvclass">[], "Hyper_State_Machine out"=w934:refnum<class "Commander.lvclass">)  [unwired: 5 in, 2 out]
        n274 = Build Array (concatenate)(w934, w932) -> (w937:refnum<class "State_Interface.lvclass">[])
        n275 = for {
          tunnel: T2 {"Command"="Exit", "Data"=variant} ("State") -> [w944]
          tunnel: w937 -> [w943] mode=indexing
          tunnel: refnum<class "Hyper_State_Machine.lvclass"> refnum ("SSW_Hyper_State_Machine.lvlibp:Hyper_State_Machine.lvclass") -> [w941]
          tunnel: w931 -> [w940]
          n276 = To More Specific Class(target class=w941, reference=w943, error in=w940) -> (specific class reference=w942:refnum<class "Hyper_State_Machine.lvclass">)  [unwired: 1 out]
          n277 = call-dynamic "State_LIFO.vi"("State_Interval(Enable)"=FALSE, "State Machine"=w944, "State_Machine_Class in"=w942) -> ()  [unwired: 7 in, 2 out]
        }
      }
    }
  }
  n278 = call-dynamic "Get_Child_State.vi"("error in (no error)"=w14, "Hyper_State_Machine in"=w15) -> ("error out"=w10:errorcluster, "Child_State"=w13:refnum<class "State_Interface.lvclass">[], "Hyper_State_Machine out"=w11:refnum<class "Commander.lvclass">)  [unwired: 5 in, 2 out]
  n279 = Build Array (concatenate)(w11, w13) -> (w12:refnum<class "State_Interface.lvclass">[])
  n280 = Merge Errors(w10, w6, w5, w4, w3, w2, w1) -> (w7:errorcluster)
  n281 = for {
    tunnel: w12 -> [w951] mode=indexing
    tunnel: refnum<class "Hyper_State_Machine.lvclass"> refnum ("SSW_Hyper_State_Machine.lvlibp:Hyper_State_Machine.lvclass") -> [w947]
    shift-right: [w946] -> w8
    shift-left: w7 -> [w949]
    n282 = To More Specific Class(target class=w947, reference=w951, error in=w949) -> (specific class reference=w950:refnum<class "Hyper_State_Machine.lvclass">, error out=w948:errorcluster)
    n283 = call-dynamic "State_Destroy.vi"("error in (no error)"=w948, "State_Machine_Class in"=w950) -> ("error out"=w946:errorcluster)  [unwired: 9 in]
  }
  n284 = call <vilib>:"Simple Error Handler.vi"("error in (no error)"=w8) -> ()  [unwired: 4 in, 5 out]
